vi "Oxford-1820-Main_.vi"() -> ()   [LabVIEW 2016]
uses:
  <instrlib>/Mercury iXX/Public/Controls/Unit String.ctl
  <instrlib>/Mercury iXX/Public/Libraries/Temperature/Controls/Temperature Device (Read).ctl
  <instrlib>/Mercury iXX/Public/Controls/Manufacturing Data.ctl
  <instrlib>/Mercury iXX/Public/Libraries/Temperature/Controls/Temperature Sensor Type.ctl
  <instrlib>/Mercury iXX/Public/Libraries/Temperature/Controls/Excitation Cluster.ctl
  <instrlib>/Mercury iXX/Public/Libraries/Temperature/Controls/Excitation Type.ctl
  <instrlib>/Mercury iXX/Public/Libraries/Temperature/Controls/Calibration Cluster.ctl
  <instrlib>/Mercury iXX/Public/Libraries/Temperature/Controls/Calibration Interpolation.ctl
  <instrlib>/Mercury iXX/Public/Libraries/Temperature/Controls/Loop Cluster.ctl
  <instrlib>/Mercury iXX/Public/Libraries/Temperature/Controls/Temperature Signals Cluster.ctl
  <instrlib>/Mercury iXX/Public/Libraries/Heater/Controls/Heater Device (Read).ctl
  <instrlib>/Mercury iXX/Public/Libraries/Heater/Controls/Heater Signals Cluster.ctl
  <instrlib>/Mercury iXX/Public/Libraries/Level Meter/Controls/Level Meter (Read).ctl
  <instrlib>/Mercury iXX/Public/Libraries/Level Meter/Controls/Nitrogen Configuration.ctl
  <instrlib>/Mercury iXX/Public/Libraries/Level Meter/Controls/Frequency Configuration.ctl
  <instrlib>/Mercury iXX/Public/Libraries/Level Meter/Controls/Signals.ctl
  <instrlib>/Mercury iXX/Public/Libraries/Level Meter/Controls/Helium Configuration.ctl
  <instrlib>/Mercury iXX/Public/Libraries/Level Meter/Controls/Resistance Configuration.ctl
  <instrlib>/Mercury iXX/Public/Libraries/Level Meter/Controls/Pre-Pulse.ctl
  <instrlib>/Mercury iXX/Public/Libraries/Level Meter/Controls/Pulse.ctl
  <instrlib>/Mercury iXX/Public/Libraries/Auxiliary/Controls/AUX Device (Read).ctl
  <instrlib>/Mercury iXX/Public/Libraries/Auxiliary/Controls/AUX Signals (Read).ctl
  <instrlib>/Mercury iXX/Public/Libraries/Magnet/Controls/Device (Read).ctl
  <instrlib>/Mercury iXX/Public/Libraries/Magnet/Controls/Signals (Read).ctl
  <instrlib>/Mercury iXX/Public/Libraries/Magnet/Controls/Identifier.ctl
  <instrlib>/Mercury iXX/Public/Libraries/Pressure/Controls/Pressure Device (Read).ctl
  <instrlib>/Mercury iXX/Public/Libraries/Pressure/Controls/Pressure Sensor Type.ctl
  <instrlib>/Mercury iXX/Public/Libraries/Pressure/Controls/Calibration Cluster.ctl
  <instrlib>/Mercury iXX/Public/Libraries/Pressure/Controls/Calibration Interpolation.ctl
  <instrlib>/Mercury iXX/Public/Libraries/Pressure/Controls/Loop Cluster.ctl
  <instrlib>/Mercury iXX/Public/Libraries/Pressure/Controls/Pressure Signals Cluster.ctl
  <instrlib>/Mercury iXX/Mercury iXX.lvlib
  <instrlib>/Mercury iXX/Public/Controls/Comms Transport Layer.ctl
  <instrlib>/Mercury iXX/Public/Libraries/Pressure/Open/Open Pressure Device.vi
  <instrlib>/Mercury iXX/Public/Libraries/Pressure.lvlib
  <instrlib>/Mercury iXX/Public/Libraries/Pressure/Configuration/Read/Pressure Device (Read).vi
  <instrlib>/Mercury iXX/Public/Libraries/System/Read/Display Automatic Dimming (Read).vi
  <instrlib>/Mercury iXX/Public/Libraries/System.lvlib
  <instrlib>/Mercury iXX/Public/Libraries/System/Read/Display Automatic Dimming Time (Read).vi
  <instrlib>/Mercury iXX/Public/Libraries/System/Read/Display Brightness (Read).vi
  <instrlib>/Mercury iXX/Public/Libraries/System/Read/Mode (Read).vi
  <instrlib>/Mercury iXX/Public/Libraries/System/Read/Serial Number (Read).vi
  <instrlib>/Mercury iXX/Public/Libraries/System/Read/FVer (Read).vi
  <instrlib>/Mercury iXX/Public/Libraries/System/Read/HVer (Read).vi
  <instrlib>/Mercury iXX/Public/Libraries/System/Set/DateTime (Set).vi
  <instrlib>/Mercury iXX/Public/Libraries/Control Loop/Configuration/Read/Control Loop (Read).vi
  <instrlib>/Mercury iXX/Public/Libraries/Control Loop.lvlib
  <instrlib>/Mercury iXX/Public/Libraries/Heater/Configuration/Read/Maximum Power (Read).vi
  <instrlib>/Mercury iXX/Public/Libraries/Heater.lvlib
  <instrlib>/Mercury iXX/Public/Libraries/Heater/Configuration/Read/Nominal Resistance (Read).vi
  <instrlib>/Mercury iXX/Public/Libraries/Temperature/Signals/Read/Temperature (Read).vi
  <instrlib>/Mercury iXX/Public/Libraries/Temperature.lvlib
  <instrlib>/Mercury iXX/Public/Libraries/Pressure/Signals/Read/Current (Read).vi
  <instrlib>/Mercury iXX/Public/Libraries/Temperature/Configuration/Read/Calibration Cold Limit (Read).vi
  <instrlib>/Mercury iXX/Public/Libraries/Temperature/Configuration/Read/Calibration Hot Limit (Read).vi
  <instrlib>/Mercury iXX/Public/Libraries/Temperature/Configuration/Read/Excitation Type (Read).vi
  <instrlib>/Mercury iXX/Public/Libraries/Temperature/Configuration/Read/Temperature Sensor (Read).vi
  <instrlib>/Mercury iXX/Public/Libraries/Temperature/Configuration/Read/Temperature Device (Read).vi
  <instrlib>/Mercury iXX/Public/Libraries/Temperature/Configuration/Read/Nickname (Read).vi
  <instrlib>/Mercury iXX/Public/Libraries/Temperature/Configuration/Read/Excitation Magnitude (Read).vi
  <instrlib>/Mercury iXX/Public/Libraries/Temperature/Configuration/Read/Serial Number (Read).vi
  <instrlib>/Mercury iXX/Public/Libraries/System/Read/Catalogue (Read).vi
  <instrlib>/Mercury iXX/Public/Libraries/System/Read/Flash Space (Read).vi
  <instrlib>/Mercury iXX/Public/Libraries/System/Read/DateTime (Read).vi
  <instrlib>/Mercury iXX/Public/Libraries/System/Read/Time (Read).vi
  <instrlib>/Mercury iXX/Public/Libraries/System/Read/Date (Read).vi
  <instrlib>/Mercury iXX/Public/Libraries/System/Open/Open System.vi
  <instrlib>/Mercury iXX/Public/Libraries/Temperature/Open/Open Temperature Device.vi
  <instrlib>/Mercury iXX/Public/Libraries/Pressure/Signals/Read/Voltage (Read).vi
  <instrlib>/Mercury iXX/Public/Libraries/Auxiliary/Open/Open Auxiliary Device.vi
  <instrlib>/Mercury iXX/Public/Libraries/Auxiliary.lvlib
  <instrlib>/Mercury iXX/Public/Libraries/Auxiliary/Signals/Read/Percent Open (Read).vi
  <instrlib>/Mercury iXX/Public/Libraries/Auxiliary/Configuration/Read/Temperature Error Sensitivity (Read).vi
  <instrlib>/Mercury iXX/Public/Libraries/Auxiliary/Configuration/Read/Valve Gearing (Read).vi
  <instrlib>/Mercury iXX/Public/Libraries/Auxiliary/Configuration/Read/Temperature Error Voltage Sensitivity (Read).vi
  <instrlib>/Mercury iXX/Public/Libraries/Magnet/Configuration/Read/Current to Field Factor (Read).vi
  <instrlib>/Mercury iXX/Public/Libraries/Magnet.lvlib
  <instrlib>/Mercury iXX/Public/Libraries/Magnet/Open/Open Magnet Device.vi
  <instrlib>/Mercury iXX/Public/Libraries/Magnet/Configuration/Read/PSU Action Status (Read).vi
  <instrlib>/Mercury iXX/Public/Libraries/Magnet/Configuration/Read/Magnet Device (Read).vi
  <instrlib>/Mercury iXX/Public/Libraries/Magnet/Configuration/Read/Switch Present (Read).vi
  <instrlib>/Mercury iXX/Public/Libraries/Temperature/Signals/Read/Voltage (Read).vi
  <instrlib>/Mercury iXX/Private/Controls/Query Dynamic Reference.ctl
  <instrlib>/Mercury iXX/Public/Controls/Mercury Reference.ctl
  <instrlib>/Mercury iXX/Public/Libraries/Level Meter/Open/Open Level Meter Device.vi
  <instrlib>/Mercury iXX/Public/Libraries/Level Meter.lvlib
  <instrlib>/Mercury iXX/Public/Libraries/Level Meter/Signals/Read/Probe Level Nitrogen (Read).vi
  <instrlib>/Mercury iXX/Public/Libraries/Level Meter/Configuration/Read/Nitrogen Freq at 100 (Read).vi
  <instrlib>/Mercury iXX/Public/Libraries/Level Meter/Signals/Read/Probe Level Helium (Read).vi
  <instrlib>/Mercury iXX/Public/Libraries/Level Meter/Signals/Read/Probe Resistance Helium (Read).vi
  <instrlib>/Mercury iXX/Public/Libraries/Level Meter/Configuration/Read/Nitrogen Pulse Count Period (Read).vi
  <instrlib>/Mercury iXX/Public/Libraries/Magnet/Signals/Read/Switch Heater Status (Read).vi
  <instrlib>/Mercury iXX/Public/Libraries/Magnet/Signals/Read/Current (Read).vi
  <instrlib>/Mercury iXX/Public/Libraries/Magnet/Configuration/Set/PSU Action Status (Set).vi
  <instrlib>/Mercury iXX/Public/Libraries/Magnet/Controls/PSU Actions.ctl
  <instrlib>/Mercury iXX/Public/Libraries/Magnet/Signals/Set/Target Field Rate (Set).vi
  <instrlib>/Mercury iXX/Public/Libraries/Magnet/Signals/Read/Persistant Field (Read).vi
  <instrlib>/Mercury iXX/Public/Libraries/Magnet/Signals/Read/Target Field (Read).vi
  <instrlib>/Mercury iXX/Public/Libraries/Magnet/Signals/Set/Target Field (Set).vi
  <instrlib>/Mercury iXX/Public/Libraries/Magnet/Configuration/Read/Software Voltage Limit (Read).vi
  <instrlib>/Mercury iXX/Public/Controls/ISOBus Address.ctl
  <instrlib>/Mercury iXX/Public/Libraries/Heater/Signals/Read/Power (Read).vi
  <instrlib>/Mercury iXX/Public/Libraries/Heater/Signals/Read/Voltage (Read).vi
  <instrlib>/Mercury iXX/Public/Libraries/Auxiliary/Signals/Read/Position (Read).vi
  <instrlib>/Mercury iXX/Public/Libraries/Auxiliary/Configuration/Read/Stepper Speed (Read).vi
  <instrlib>/Mercury iXX/Public/Libraries/Level Meter/Signals/Read/Probe Count Nitrogen (Read).vi
  <instrlib>/Mercury iXX/Public/Libraries/Magnet/Signals/Read/Current Rate (Read).vi
  <instrlib>/Mercury iXX/Public/Libraries/Lambda/Configuration/Set/Lambda Percentage Flow (Set).vi
  <instrlib>/Mercury iXX/Public/Libraries/Lambda.lvlib
  <instrlib>/Mercury iXX/Public/Libraries/Lambda/Open/Open Lambda Device.vi
  <instrlib>/Mercury iXX/Public/Libraries/Lambda/Configuration/Set/Lambda Flow Auto (Set).vi
  <instrlib>/Mercury iXX/Public/Libraries/Level Meter/Configuration/Set/Pulse Slow-Fast (Set).vi
  <instrlib>/Mercury iXX/Public/Controls/Response String.ctl
  <instrlib>/Mercury iXX/Public/Libraries/Temperature/Signals/Read/Resistance (Read).vi
  <instrlib>/Mercury iXX/Public/Libraries/Magnet/Signals/Read/Persistant Current (Read).vi
  <userlib>/_OpenG.lib/error/error.llb/Filter Error Codes (Array)__ogtk.vi
  <instrlib>/Mercury iXX/Public/Libraries/Heater/Configuration/Read/Nickname (Read).vi
  <instrlib>/Mercury iXX/Public/Libraries/Heater/Configuration/Read/Voltage Limit (Read).vi
  <instrlib>/Mercury iXX/Public/Libraries/Heater/Configuration/Read/Serial Number (Read).vi
  <instrlib>/Mercury iXX/Public/Libraries/Heater/Configuration/Read/Heater Device (Read).vi
  <instrlib>/Mercury iXX/Public/Libraries/Heater/Open/Open Heater Device.vi
  <instrlib>/Mercury iXX/Public/Libraries/Auxiliary/Configuration/Read/Gas Flow Scaling (Read).vi
  <instrlib>/Mercury iXX/Public/Libraries/Auxiliary/Configuration/Read/Minimum Gas Flow (Read).vi
  <instrlib>/Mercury iXX/Public/Libraries/Auxiliary/Configuration/Read/Serial Number (Read).vi
  <instrlib>/Mercury iXX/Public/Libraries/Auxiliary/Configuration/Read/Aux Device (Read).vi
  <instrlib>/Mercury iXX/Public/Libraries/Pressure/Configuration/Read/Nickname (Read).vi
  <instrlib>/Mercury iXX/Public/Libraries/Level Meter/Configuration/Read/Helium Pulse Duration (Read).vi
  <instrlib>/Mercury iXX/Public/Libraries/Level Meter/Configuration/Read/Helium Pulse Mag (Read).vi
  <instrlib>/Mercury iXX/Public/Libraries/Level Meter/Configuration/Read/Helium Probe Resistance (Read).vi
  <instrlib>/Mercury iXX/Public/Libraries/Level Meter/Configuration/Read/Serial Number (Read).vi
  <instrlib>/Mercury iXX/Public/Libraries/Level Meter/Configuration/Read/Level Meter Device (Read).vi
  <instrlib>/Mercury iXX/Public/Libraries/Magnet/Configuration/Read/Current Limit (Read).vi
  <instrlib>/Mercury iXX/Public/Libraries/Magnet/Configuration/Read/Output Configuration (Read).vi
  <instrlib>/Mercury iXX/Public/Libraries/Magnet/Configuration/Read/Bipolar Output (Read).vi
  <instrlib>/Mercury iXX/Public/Libraries/Magnet/Configuration/Read/Serial Number (Read).vi
  <instrlib>/Mercury iXX/Public/Libraries/Magnet/Signals/Read/Target Field Rate (Read).vi
  <instrlib>/Mercury iXX/Public/Libraries/Magnet/Signals/Read/Field (Read).vi
  <instrlib>/Mercury iXX/Public/Libraries/Magnet/Signals/Read/Voltage (Read).vi
  <instrlib>/Mercury iXX/Public/Libraries/Heater/Signals/Read/Current (Read).vi
  <instrlib>/Mercury iXX/Public/Libraries/Magnet/Controls/Switch Heater.ctl
  <instrlib>/Mercury iXX/Public/Libraries/Magnet/Signals/Set/Switch Heater Status (Set).vi
panel:
  in  "Tab Control 6":enum32{"Page 1", "Page 2"}(tab)
  in  "Tab Control 5":enum32{"Page 1", "Page 2"}(tab)
  in  "Open Needle Valve":bool
  in  "Close Needle Valve":bool
  in  "Lambda":bool
  out "LPF NV (%)":dbl format="%_6g"
  out "LPF Pressure":dbl format="%_5f mB"
  out "Magnet Field (T) 2":dbl(knob) caption="Voltage (V)" scale=-20.0..20.0
  out "Voltage (V) 2":dbl(knob)=-0.0003 caption="Voltage (V)" scale=-10.0..10.0
  out "Current (A)":dbl(knob)=0.0006 scale=-180.0..180.0
  in  "Tab Control 4":enum32{"Page 1", "Page 2"}(tab)
  out "N2 LEVEL":dbl=61.3025 format="%.0f %"
  out "He LVL Chart":dbl(slide)=52.0833 scale=0.0..100.0
  out "N2 LVL Chart":dbl(slide)=61.3025 scale=0.0..100.0
  out "He LEVEL 3":dbl=61.3025 format="%.0f %"
  in  "Fast/Slow Fill":bool
  in  "Tab Control 3":enum32{"Page 1", "Page 2"}(tab)
  out "Magnet T":dbl=3.8705 format="%_2f K"
  out "Magnet R":dbl=3.8705 format="%_3f ohms"
  out "LPF R":dbl=4.2075 format="%_3f ohms"
  out "Voltage (V)":dbl=-0.0003 format="%.5f"
  out "LPF T":dbl=4.2075 format="%_2f K"
  out "Current (A)":dbl=0.0006 format="%.5f"
  out "Magnet Status 2":string
  in  "Tab Control 2":enum32{"Page 1", "Page 2"}(tab)
  in  "Hold":bool
  in  "To Set":bool
  in  "Send to IPS":bool
  out "Power Supply Field (T)":dbl=0.0001 format="%#.5f"
  in  "Target Field (T) 2":dbl format="%#.5f"
  out "Target Field (T)":dbl format="%#.5f"
  in  "Target Rate (T/min)":dbl=0.1 format="%.5f"
  out "Target  Rate (T/min)":dbl=1.0 format="%.5f"
  out "Magnet Field (T)":dbl format="%.5f"
  out "He LEVEL":dbl=52.0833 format="%.0f %"
  in  "PS Heat":bool
  out "Switch Time":string="11:11:48"
  in  "To Zero":bool
  in  "Clamp":bool
  in  "Toolbar":enum32{"Page 1", "Page 2"}(tab)
  in  "Start 2":bool
  in  "Stop 2":bool
  in  "Minimize":bool
  out "ETA":string
  out "Magnet Status 3":string="Clamped"
  in  "Remote Mode":bool
  out "Sentinel":bool=TRUE
  out "SWITCH HEATER":bool
  out "LPF ON":timestamp
  in  "Tab Control":T1(tab)
  in  "Mercury Functions":T2(tab)=enum."Temperature"
  out "time stamp":timestamp=timestamp(3543841780 s since 1904-01-01)
  out "Free Space":i32=166384 caption="Free Space (KB)"
  out "Set Date Response":string="VALID"
  out "String":string="NORM" caption="User Mode"
  out "Date":string="2016:04:18"
  out "Time":string="11:29:40"
  out "Hardware Version":string="65"
  out "Firmware Version":string="2.2.6.20"
  out "Serial Number":string="154650110"
  out "ITC Devices":string[](array[string])=["DB4.G1:AUX", "DB8.P1:PRES", "MB0.H1:HTR", "MB1.T1:TEMP"]
  out "S/W Version(s)":string[](array[string])=["2.2.6.20\n"]
  out "Serial Number(s)":string[](array[string])=["154650110"]
  out "# of Instruments":i32=1
  out "Automatic Dimming":string="OFF"
  out "Dimming Time":string="5"
  out "Display Brightness":string="100"
  in  "ITC IP Address":string="130.49.180.101"
  out "Excitation Magnitude":dbl=5.0
  out "Sensor Type":string="NTC"
  out "Excitation Type":string="UNIP"
  out "Hot Limit":dbl=1000.0
  out "H Unit":T3="K"
  out "Cold Limit":dbl=1000.0
  out "C Unit":T3="K"
  out "Unit":T3
  out "Voltage":dbl=0.005
  out "V Unit":T3="V"
  out "Temperature":dbl=4.2075
  out "T Unit":T3="K"
  out "Temperature Device Settings":T4={"Manufacturing"={"Hardware Version"="65", "Firmware Version"="2.2", "Serial Number"="154650110"}, "Temperature Sensor Type"="NTC", "Excitation"={"Excitation Type"="UNIP", "Magnitude"="5.00"}, "Calibration"={"Filename"="59543_iTC-lambda.dat", "Interpolation"="LIN", "Scaling Factor"="1", "Offset Factor"="0", "Hot Limit"="1000.00K", "Cold Limit"="1000.00K", "Last Calibration"="", "Reference"="Internal"}, "Control Loop"={"Heater"="", "Auxiliary"="", "Heater Auto"="", "Percentage Heat"="", "Temperature Set Point"="", "PID Auto (from file)"="", "P Value"="", "I Value"="", "D Value"="", "Auto PID Table Filename"="", "Flow Auto"="", "Target Heater Table"="", "Sweep mode"="", "Sweep Table Filename"="", "Percentage Flow"=""}, "Temperature Signals"={"Voltage"="5.0000mV", "Current"="3.9694µA", "Power"="0.0199µW", "Resistance"="1259.6510R", "Temperature"="4.2075K", "Sensitivity"="299.3801R/K", "Reference"="N/A"}, "Nickname"="Mag_AB_MB1", "Status"="0"}
  out "Temp S/N":string="154650110"
  out "T Nickname":string="Mag_AB_MB1"
  out "T Loop Details":T11
  out "Heater Device Settings":T13={"Manufacturing"={"Hardware Version"="65", "Firmware Version"="2.3", "Serial Number"="154650110"}, "Nickname"="MB0.H1", "Voltage Limit"="1", "Nominal Resistance"="10", "Maximum Power"="0.1000", "Heater Signals"={"Voltage"="0.0507V", "Current"="-0.0000A", "Power"="0.0000W"}, "Status"="2"}
  out "Htr C Unit":T3="A"
  out "Htr P Unit":T3="W"
  out "Htr V Unit":T3="V"
  out "Htr Current":dbl=-0.0
  out "Htr Power":dbl
  out "Htr Voltage":dbl=0.0507
  out "Power Unit":T3
  out "Volt Unit":T3
  out "Res Unit":T3
  out "Maximum Power":dbl=0.1
  out "Htr Resistance":dbl=10.0
  out "Htr Voltage Limit":dbl=1.0
  out "Htr S/N":string="154650110"
  out "Htr Nickname":string="MB0.H1"
  out "Pressure Device":T15={"Manufacturing"={"Hardware Version"="3", "Firmware Version"="1.10", "Serial Number"="151150091"}, "Temperature Sensor Type"="RAT", "Calibration"={"Filename"="Lambda pressure control_10V ratiometric.dat", "Interpolation"="LIN", "Scaling Factor"="1", "Offset Factor"="-0.0004", "High Limit"="1000.00K", "Low Limit"="1000.00K", "Last Calibration"=""}, "Control Loop"={"Heater"="None", "Auxiliary"="None", "Heater Auto"="", "Percentage Heat"="", "Pressure Set Point"="", "PID Auto (from file)"="", "P Value"="", "I Value"="", "D Value"="1.0", "Auto PID Table Filename"="", "Flow Auto"="", "Target Heater Table"="", "Sweep mode"="", "Sweep Table Filename"="", "Percentage Flow"=""}, "Pressure Signals"={"Voltage"="-0.0822mV", "Current"="-0.0000A", "Power"="0.0000W", "Pressure"="0.0000mB"}, "Nickname"="Lam_P_DB8", "Status"="0"}
  out "Nickname":string="Lam_P_DB8"
  out "Current":dbl=-0.0
  out "Voltage":dbl=-8.219999999999999e-05
  out "Auxiliary Device Details":T21={"Manufacturing"={"Hardware Version"="65", "Firmware Version"="3.1", "Serial Number"="154650084"}, "Min Flow"=0.0, "Scaling Factor"=50.0, "Temp Err"=9.0, "Temp V Err"=11.0, "Gear"=2, "Speed"=2, "Signals"={"Position"=0.0, "% Open"=0.0, "I0"="ON", "I1"="OFF", "I2"="OFF", "I3"="OFF", "O0"="OFF", "O1"="OFF", "O2"="OFF", "O3"="OFF"}, "Nickname"="DB4.G1", "Status"="0"} {"Signals"."% Open" min=0.0 max=100.0 step=0.1 format="%.4f"; "Signals"."Position" max=20.0 step=1.0 format="%.4f"; "Speed" max=7 step=1; "Gear" max=7 step=1; "Temp V Err" min=0.0 max=20.0 step=0.1; "Temp Err" min=0.0 max=20.0 step=0.1; "Scaling Factor" min=0.0 max=99.0 step=0.1; "Min Flow" min=0.0 max=20.0 step=0.1}
  out "Aux S/N":string="154650084"
  out "Min Flow":dbl caption="Minimum Gas Flow" format="%#.1f"
  out "Scaling Factor":dbl=50.0 caption="Gas Flow Scaling Factor" format="%#.1f"
  out "Temp Err":dbl=9.0 caption="Temperature Error Sensitivity" format="%#.1f"
  out "Temp V Err":dbl=11.0 caption="Temperature Voltage Error Sensitivity" format="%#.1f"
  out "Gear":u32=2 caption="Valve Gearing"
  out "Speed":u32=2 caption="Stepper Speed"
  out "Unit 2":T3
  out "Unit 3":T3
  out "Unit 4":T3
  out "Unit 5":T3
  out "Unit 6":T3
  out "Unit 7":T3
  out "Position":u32
  out "% Open":dbl caption="Percentage Open (%)"
  out "Unit":T3
  out "Unit":T3="%"
  out "time stamp 2":timestamp=timestamp(3543841781 s since 1904-01-01)
  out "Free Space 2":i32=166316 caption="Free Space (KB)"
  out "Set Date Response 2":string="VALID"
  out "String 2":string="NORM" caption="User Mode"
  out "Date 2":string="2016:04:18"
  out "Time 2":string="11:29:45"
  out "Hardware Version 2":string="65"
  out "Firmware Version 2":string="2.2.6.20"
  out "Serial Number 2":string="153350063"
  out "IPS Devices":string[](array[string])=["DB3.L1:LVL", "GRPX:PSU", "GRPY:PSU", "GRPZ:PSU", "MB1.T1:TEMP", "PSU.M1:PSU", "PSU.M2:PSU", "PSU.M3:PSU"]
  out "S/W Version(s) 2":string[](array[string])=["2.2.6.20\n"]
  out "Serial Number(s) 2":string[](array[string])=["153350063"]
  out "# of Instruments 2":i32=1
  out "Automatic Dimming 2":string="OFF"
  out "Dimming Time 2":string="5"
  out "Display Brightness 2":string="100"
  in  "IPS IP Address":string="130.49.180.102"
  out "LVL Device DetailSettings":T23={"Manufacturing"={"Hardware Version"="65", "Firmware Version"="2.2", "Serial Number"="152450013"}, "Nitrogen Configuration"={"Frequency Configuration"={"Freq 0%"=0.0, "Freq 100%"=0.0}, "Pulse Period"=0.0}, "Signals"={"Helium Signals"={"Resistance"=75.5626, "Level"=52.0833}, "Nitrogen Signals"={"Count"=8800.0, "Freq"=487361.0, "Level"=61.3445}}, "Nickname"="DB3.L1", "Status"="0", "Helium Configuration"={"Resistance Configuration"={"Res 0%"=0.0, "Res 100%"=0.0}, "Pre-Pulse"={"Magnitude"=0.0, "Duration"=0.0}, "Pulse"={"Magnitude"=0.0, "Duration"=0.0, "Delay"=0.0}}}
  out "LVL S/N":string="152450013"
  out "LVL P Magnitude":dbl=125.0 caption="Pulse Magnitude (mA)"
  out "LVL P Duration":dbl=5.0 caption="Pulse Duration (s)"
  out "N Freq 100%":dbl=7880.0 caption="Frequency at 100% (Hz)"
  out "N Pulse Period":dbl=1000.0 caption="Pulse Period (ms)"
  out "He Res Config":T28={"Res 0%"=149.0, "Res 100%"=8.0}
  out "He Resistance":dbl=75.5626 caption="Resistance (Ohms)"
  out "He Level":dbl=52.0833 caption="Helium Level (%)"
  out "N Counter":u32 caption="Counter"
  out "N Level":dbl=61.3445 caption="Nitrogen Level (%)"
  out "Excitation Magnitude 2":dbl=5.0
  out "Sensor Type 2":string="NTC"
  out "Excitation Type 2":string="UNIP"
  out "Hot Limit 2":dbl=1000.0
  out "H Unit 2":T3="K"
  out "Cold Limit 2":dbl=1000.0
  out "C Unit 2":T3="K"
  out "Unit 12":T3
  out "Voltage 2":dbl=0.005
  out "V Unit 2":T3="V"
  out "Temperature 2":dbl=3.8706
  out "T Unit 2":T3="K"
  out "Temperature Device Settings 2":T4={"Manufacturing"={"Hardware Version"="65", "Firmware Version"="2.2", "Serial Number"="153350063"}, "Temperature Sensor Type"="NTC", "Excitation"={"Excitation Type"="UNIP", "Magnitude"="5.00"}, "Calibration"={"Filename"="Bob.dat", "Interpolation"="LIN", "Scaling Factor"="1", "Offset Factor"="0", "Hot Limit"="1000.00K", "Cold Limit"="1000.00K", "Last Calibration"="", "Reference"="Internal"}, "Control Loop"={"Heater"="", "Auxiliary"="", "Heater Auto"="", "Percentage Heat"="", "Temperature Set Point"="", "PID Auto (from file)"="", "P Value"="", "I Value"="", "D Value"="", "Auto PID Table Filename"="", "Flow Auto"="", "Target Heater Table"="", "Sweep mode"="", "Sweep Table Filename"="", "Percentage Flow"=""}, "Temperature Signals"={"Voltage"="5.0000mV", "Current"="3.5897µA", "Power"="0.0179µW", "Resistance"="1392.8897R", "Temperature"="3.8706K", "Sensitivity"="359.8580R/K", "Reference"="N/A"}, "Nickname"="MB1.T1", "Status"="0"}
  out "Temp S/N 2":string="153350063"
  out "T Nickname 2":string="MB1.T1"
  out "T Loop Details 2":T11
  out "Magnet Device Details":T31={"Manufacturing"={"Hardware Version"="NOT_FOUND", "Firmware Version"="NOT_FOUND", "Serial Number"="NOT_FOUND"}, "Nickname"="GRPZ", "Bipolar Output"="ON", "String"="PARA", "Current Limit"=174.0, "AtoB"=8.688, "Inductance"=39.406, "Switch Present"="PSU.M1", "Swh Htr Current"=86.0, "SW VLIM"=9.0, "V Trans Time"=1000.0, "Magnet PSU Signals"={"Voltage"=-0.0002, "Current"=0.0002, "Current Rate"=100.0, "Field"=0.0001, "Field Rate"=11.5101, "Persistant Current"=0.0003, "Persistant Field"=0.0, "Target Current"=0.0, "Target Field"=0.0, "Target Current Rate"=8.688, "Target Field Rate"=1.0, "Switch Heater Status (SWHT)"="OFF", "Switch Heater Status (SWHN)"="OFF"}, "PSU Action"="CLMP", "Status"="40000000", "Level Limit"=0.0, "Temperature Limit"=999.0} {"Temperature Limit" format="%#.1f"; "Level Limit" format="%#.1f"; "V Trans Time" format="%#.1f"; "SW VLIM" format="%#.1f"; "Swh Htr Current" format="%#.1f"; "Inductance" format="%#.1f"; "AtoB" format="%#.1f"; "Current Limit" format="%#.1f"}
  out "Mag S/N":string="NOT_FOUND"
  out "Bipolar Output":string="ON"
  out "Out Config":string="PARA" caption="Output Configuration"
  out "Current Limit":dbl=174.0 caption="Current Limit (A)" format="%#.1f"
  out "AtoB":dbl=8.688 caption="Current Field Factor (A/T)" format="%#.1f"
  out "Switch Present":string="PSU.M1"
  out "SW VLIM":dbl=9.0 caption="Software Voltage Limit (V)" format="%#.1f"
  out "Unit 8":T3
  out "Unit 9":T3
  out "Unit 10":T3
  out "Current Rate":dbl=100.0
  out "PSU Act Stat":string="CLMP" caption="PSU Action Status"
  out "Unit 11":T3="A/min"
  in  "Device Identifier":T33="GRPZ"
  out "Error List":T34(array[cluster])
  out "LPF on (s)":i32=5373
  # "Magnet (T)"
  # "Voltage (V)"
  # "Current (A)"
  # "Slow Rates\nCurrent Range (A)     Field Range (T)   Rate (T/min)\n0       -- 100        0    -- 11.5      0.91\n100     -- 150        11.5 -- 17.2      0.23\n150     -- 155.467    17.2 -- 18        0.11\n155.567 -- 172.471    18   -- 20        0.11\n\nFast Rates\nCurrent Range (A)     Field Range (T)   Rate (T/min)\n0       -- 155.467    0    -- 18        1.0\n155.567 -- 172.471    18   -- 20        0.25"
  # "Helium"
  # "Nitrogen"
  # "v17/02/01"
  # "ITC: 101\nIPS: 102\nIPS VR: 67"
  # "ITC: 101\nIPS: 102\nIPS VR: 67"
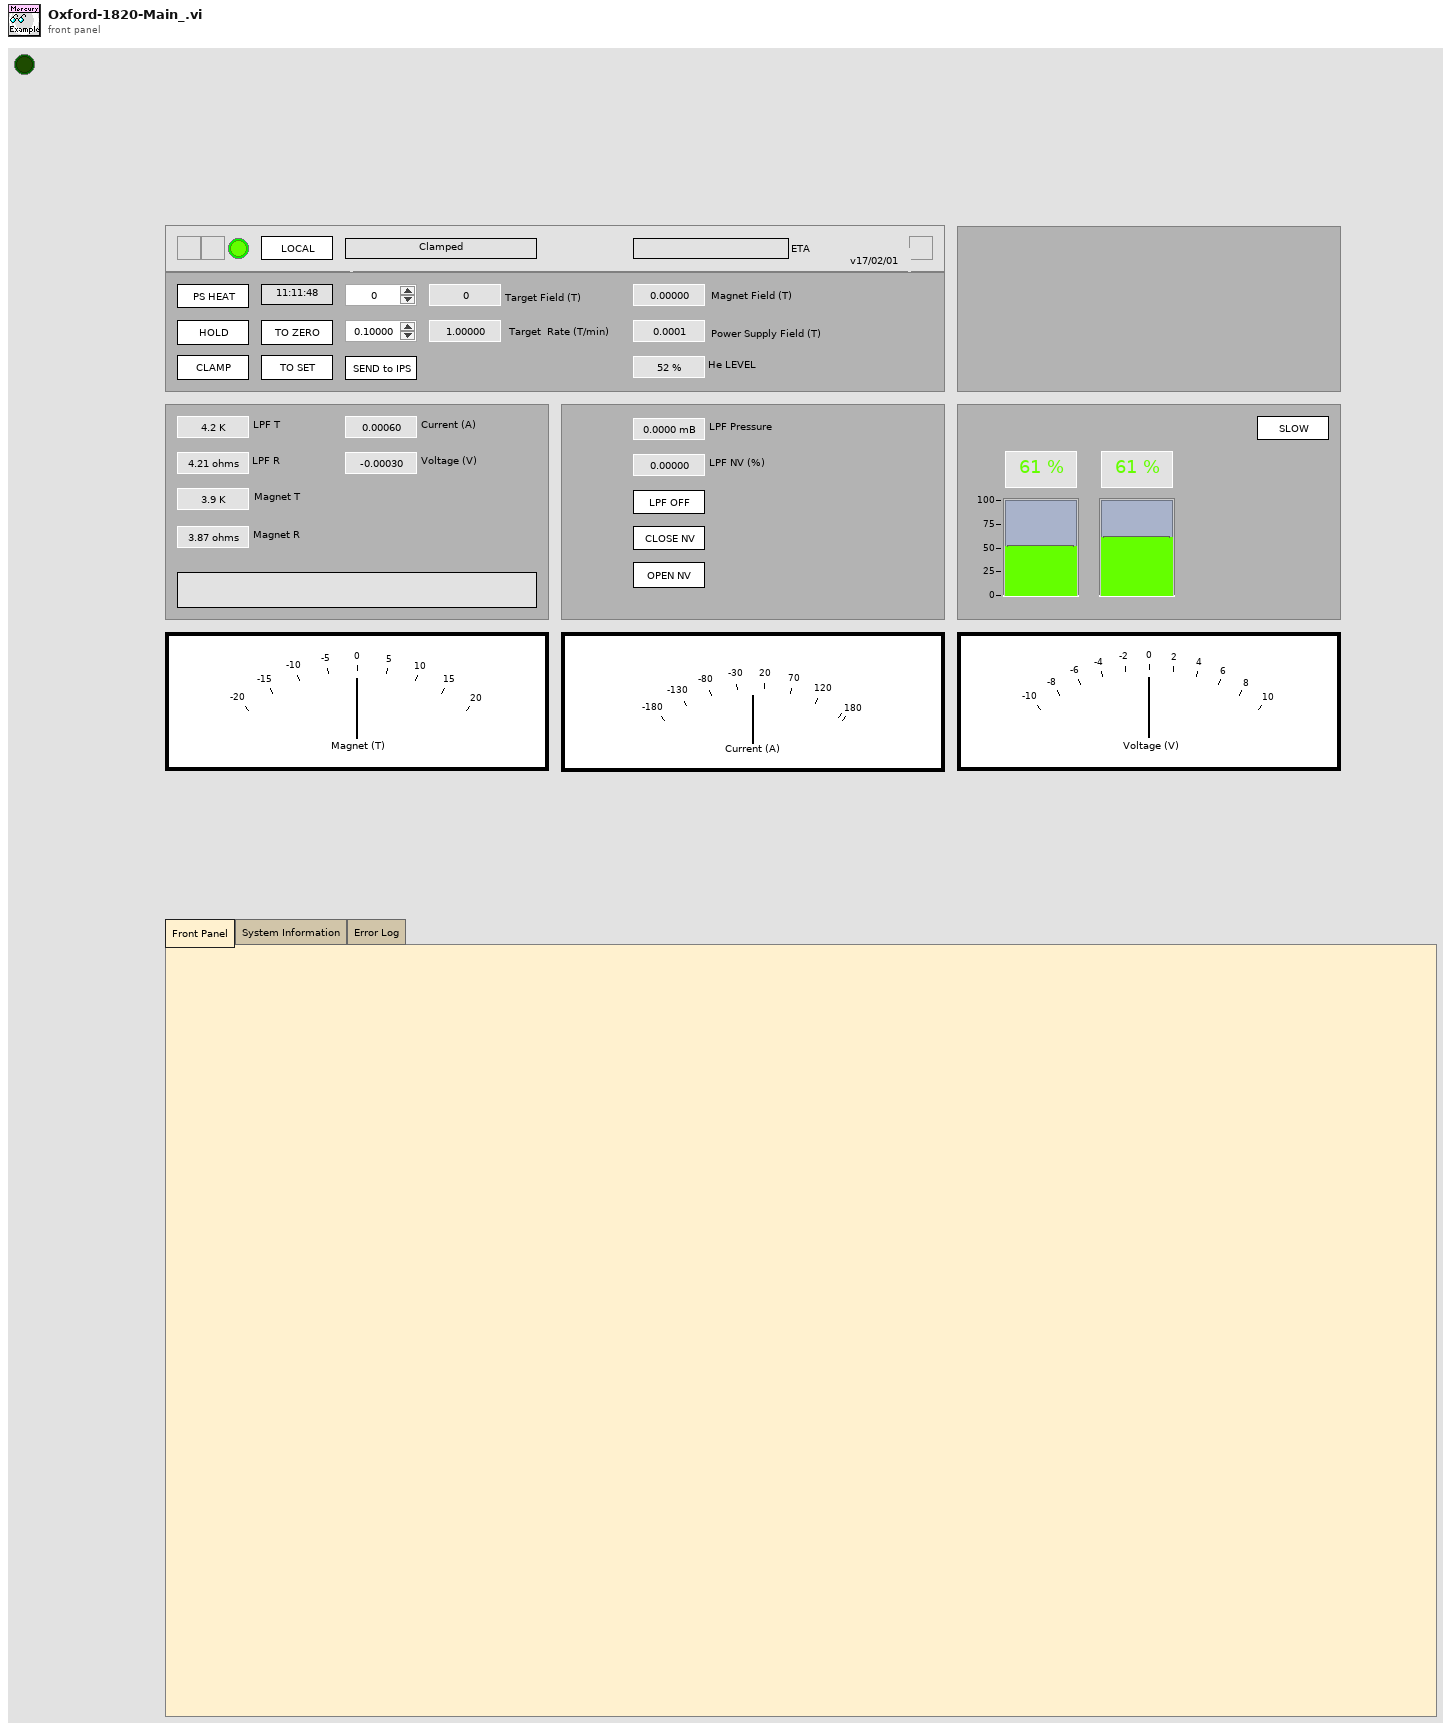
[diagram p1: front panel]
types:
  T1 = enum32{"Front Panel", "System Information", "Error Log"}
  T2 = enum32{"System: ITC", "Temperature", "Heater", "Pressure", "Auxiliary", "System: IPS", "Level Meter", "Temperature 2", "Magnet"}
  T3 = typedef "Mercury iXX.lvlib/Unit String.ctl" = string
  T4 = typedef "Mercury iXX.lvlib/Temperature.lvlib/Temperature Device (Read).ctl" = cluster{"Manufacturing":T5, "Temperature Sensor Type":T6, "Excitation":T7, "Calibration":T9, "Control Loop":T11, "Temperature Signals":T12, "Nickname":string, "Status":string}
  T5 = typedef "Mercury iXX.lvlib/Manufacturing Data.ctl" = cluster{"Hardware Version":string, "Firmware Version":string, "Serial Number":string}
  T6 = typedef "Mercury iXX.lvlib/Temperature.lvlib/Temperature Sensor Type.ctl" = string
  T7 = typedef "Mercury iXX.lvlib/Temperature.lvlib/Excitation Cluster.ctl" = cluster{"Excitation Type":T8, "Magnitude":string}
  T8 = typedef "Mercury iXX.lvlib/Temperature.lvlib/Excitation Type.ctl" = string
  T9 = typedef "Mercury iXX.lvlib/Temperature.lvlib/Calibration Cluster.ctl" = cluster{"Filename":string, "Interpolation":T10, "Scaling Factor":string, "Offset Factor":string, "Hot Limit":string, "Cold Limit":string, "Last Calibration":string, "Reference":string}
  T10 = typedef "Mercury iXX.lvlib/Temperature.lvlib/Calibration Interpolation.ctl" = string
  T11 = typedef "Mercury iXX.lvlib/Temperature.lvlib/Loop Cluster.ctl" = cluster{"Heater":string, "Auxiliary":string, "Heater Auto":string, "Percentage Heat":string, "Temperature Set Point":string, "PID Auto (from file)":string, "P Value":string, "I Value":string, "D Value":string, "Auto PID Table Filename":string, "Flow Auto":string, "Target Heater Table":string, "Sweep mode":string, "Sweep Table Filename":string, "Percentage Flow":string}
  T12 = typedef "Mercury iXX.lvlib/Temperature.lvlib/Temperature Signals Cluster.ctl" = cluster{"Voltage":string, "Current":string, "Power":string, "Resistance":string, "Temperature":string, "Sensitivity":string, "Reference":string}
  T13 = typedef "Mercury iXX.lvlib/Heater.lvlib/Heater Device (Read).ctl" = cluster{"Manufacturing":T5, "Nickname":string, "Voltage Limit":string, "Nominal Resistance":string, "Maximum Power":string, "Heater Signals":T14, "Status":string}
  T14 = typedef "Mercury iXX.lvlib/Heater.lvlib/Heater Signals Cluster.ctl" = cluster{"Voltage":string, "Current":string, "Power":string}
  T15 = typedef "Mercury iXX.lvlib/Pressure.lvlib/Pressure Device (Read).ctl" = cluster{"Manufacturing":T5, "Temperature Sensor Type":T16, "Calibration":T17, "Control Loop":T19, "Pressure Signals":T20, "Nickname":string, "Status":string}
  T16 = typedef "Mercury iXX.lvlib/Pressure.lvlib/Pressure Sensor Type.ctl" = string
  T17 = typedef "Mercury iXX.lvlib/Pressure.lvlib/Calibration Cluster.ctl" = cluster{"Filename":string, "Interpolation":T18, "Scaling Factor":string, "Offset Factor":string, "High Limit":string, "Low Limit":string, "Last Calibration":string}
  T18 = typedef "Mercury iXX.lvlib/Pressure.lvlib/Calibration Interpolation.ctl" = string
  T19 = typedef "Mercury iXX.lvlib/Pressure.lvlib/Loop Cluster.ctl" = cluster{"Heater":string, "Auxiliary":string, "Heater Auto":string, "Percentage Heat":string, "Pressure Set Point":string, "PID Auto (from file)":string, "P Value":string, "I Value":string, "D Value":string, "Auto PID Table Filename":string, "Flow Auto":string, "Target Heater Table":string, "Sweep mode":string, "Sweep Table Filename":string, "Percentage Flow":string}
  T20 = typedef "Mercury iXX.lvlib/Pressure.lvlib/Pressure Signals Cluster.ctl" = cluster{"Voltage":string, "Current":string, "Power":string, "Pressure":string}
  T21 = typedef "Mercury iXX.lvlib/Auxiliary.lvlib/AUX Device (Read).ctl" = cluster{"Manufacturing":T5, "Min Flow":dbl, "Scaling Factor":dbl, "Temp Err":dbl, "Temp V Err":dbl, "Gear":u32, "Speed":u32, "Signals":T22, "Nickname":string, "Status":string}
  T22 = typedef "Mercury iXX.lvlib/Auxiliary.lvlib/AUX Signals (Read).ctl" = cluster{"Position":dbl, "% Open":dbl, "I0":string, "I1":string, "I2":string, "I3":string, "O0":string, "O1":string, "O2":string, "O3":string}
  T23 = typedef "Mercury iXX.lvlib/Level Meter.lvlib/Level Meter (Read).ctl" = cluster{"Manufacturing":T5, "Nitrogen Configuration":T24, "Signals":T26, "Nickname":string, "Status":string, "Helium Configuration":T27}
  T24 = typedef "Mercury iXX.lvlib/Level Meter.lvlib/Nitrogen Configuration.ctl" = cluster{"Frequency Configuration":T25, "Pulse Period":dbl}
  T25 = typedef "Mercury iXX.lvlib/Level Meter.lvlib/Frequency Configuration.ctl" = cluster{"Freq 0%":dbl, "Freq 100%":dbl}
  T26 = typedef "Mercury iXX.lvlib/Level Meter.lvlib/Signals.ctl" = cluster{"Helium Signals":cluster{"Resistance":dbl, "Level":dbl}, "Nitrogen Signals":cluster{"Count":dbl, "Freq":dbl, "Level":dbl}}
  T27 = typedef "Mercury iXX.lvlib/Level Meter.lvlib/Helium Configuration.ctl" = cluster{"Resistance Configuration":T28, "Pre-Pulse":T29, "Pulse":T30}
  T28 = typedef "Mercury iXX.lvlib/Level Meter.lvlib/Resistance Configuration.ctl" = cluster{"Res 0%":dbl, "Res 100%":dbl}
  T29 = typedef "Mercury iXX.lvlib/Level Meter.lvlib/Pre-Pulse.ctl" = cluster{"Magnitude":dbl, "Duration":dbl}
  T30 = typedef "Mercury iXX.lvlib/Level Meter.lvlib/Pulse.ctl" = cluster{"Magnitude":dbl, "Duration":dbl, "Delay":dbl}
  T31 = typedef "Mercury iXX.lvlib/Magnet.lvlib/Device (Read).ctl" = cluster{"Manufacturing":T5, "Nickname":string, "Bipolar Output":string, "String":string, "Current Limit":dbl, "AtoB":dbl, "Inductance":dbl, "Switch Present":string, "Swh Htr Current":dbl, "SW VLIM":dbl, "V Trans Time":dbl, "Magnet PSU Signals":T32, "PSU Action":string, "Status":string, "Level Limit":dbl, "Temperature Limit":dbl}
  T32 = typedef "Mercury iXX.lvlib/Magnet.lvlib/Signals (Read).ctl" = cluster{"Voltage":dbl, "Current":dbl, "Current Rate":dbl, "Field":dbl, "Field Rate":dbl, "Persistant Current":dbl, "Persistant Field":dbl, "Target Current":dbl, "Target Field":dbl, "Target Current Rate":dbl, "Target Field Rate":dbl, "Switch Heater Status (SWHT)":string, "Switch Heater Status (SWHN)":string}
  T33 = typedef "Mercury iXX.lvlib/Magnet.lvlib/Identifier.ctl" = string
  T34 = cluster{"time":timestamp, "code":i32, "source":string}[]
  T35 = typedef "LVRectTypeDef.ctl" = cluster{"Left":i16, "Top":i16, "Right":i16, "Bottom":i16}
  T36 = cluster{"Hold":bool, "Clamp":bool, "To Set":bool, "To Zero":bool, "Send to IPS":bool, "PS Heat":bool, "Lambda":bool}
  T37 = typedef "Mercury iXX.lvlib/Magnet.lvlib/PSU Actions.ctl" = string
  T38 = typedef "Mercury iXX.lvlib/Magnet.lvlib/Switch Heater.ctl" = string
  T39 = typedef "Mercury iXX.lvlib/ISOBus Address.ctl" = i32
  T40 = typedef "Mercury iXX.lvlib/Response String.ctl" = string
  T41 = enum32{"invalid app kind", "Development System", "Run Time System", "Student Edition", "Embedded LabVIEW", "Evaluation", "Custom"}
  T42 = cluster{"time":timestamp, "code":i32, "source":string}
  T43 = enum32{"Invalid", "Standard", "Closed", "Hidden", "Minimized", "Maximized"}
  T44 = cluster{"Magnet Field":dbl, "PS Field":dbl, "Target Field":dbl, "Target Field Rate":dbl, "Voltage":dbl, "Current":dbl}
  T45 = typedef "Mercury iXX.lvlib/Comms Transport Layer.ctl" = enum16{"Ethernet TCP/IP", "USB", "ISOBus - RS-232", "GPIB"}
  T46 = typedef "Mercury iXX.lvlib/Query Dynamic Reference.ctl" = refnum<vi>
  T47 = typedef "Mercury iXX.lvlib/Mercury Reference.ctl" = cluster{"Comms":refnum<visa-resource-name>, "Device ID":string[], "Comms Layer":T45, "Command":string, "Query reference":T46}
  T48 = cluster{"Core":cluster{"Current VI Reference":refnum<vi>, "Close Panel on Exit?":bool}, "Mercury ITC Ref":cluster{"Comms":refnum<visa-resource-name>, "Device ID":string[], "Comms Layer":T45, "Command":string, "Query reference":T46}, "Mercury IPS Ref":T47, "sentinel":bool, "Error Log":cluster{"time":timestamp, "code":i32, "source":string}[]}
  T49 = typedef "Actions.ctl" = cluster{"Hold":bool, "Clamp":bool, "To Set":bool, "To Zero":bool, "Send to IPS":bool, "PS Heat":bool, "Lambda":bool}
  T50 = typedef "Targets.ctl" = cluster{"Target Field (T)":dbl, "Target Field Rate (T/min)":dbl}
  T51 = cluster{"Target Field (T)":dbl, "Target Field Rate (T/min)":dbl}
  T52 = cluster{"Comms":refnum<visa-resource-name>, "Device ID":string[], "Comms Layer":T45, "Command":string, "Query reference":T46}
  T53 = typedef "Filtered Error Details - Cluster__ogtk.ctl" = cluster{"code":i32, "source":string}
  T54 = cluster{"Current VI Reference":refnum<vi>, "Close Panel on Exit?":bool}
  T55 = typedef "Mercury iXX.lvlib/System.lvlib/User Mode.ctl" = string
  T56 = typedef "Mercury iXX.lvlib/Magnet.lvlib/Output Configuration.ctl" = string
  T57 = typedef "Status.ctl" = cluster{"Magnet Field":dbl, "PS Field":dbl, "Target Field":dbl, "Target Field Rate":dbl, "Voltage":dbl, "Current":dbl, "Switch":bool, "Mercury State":string}
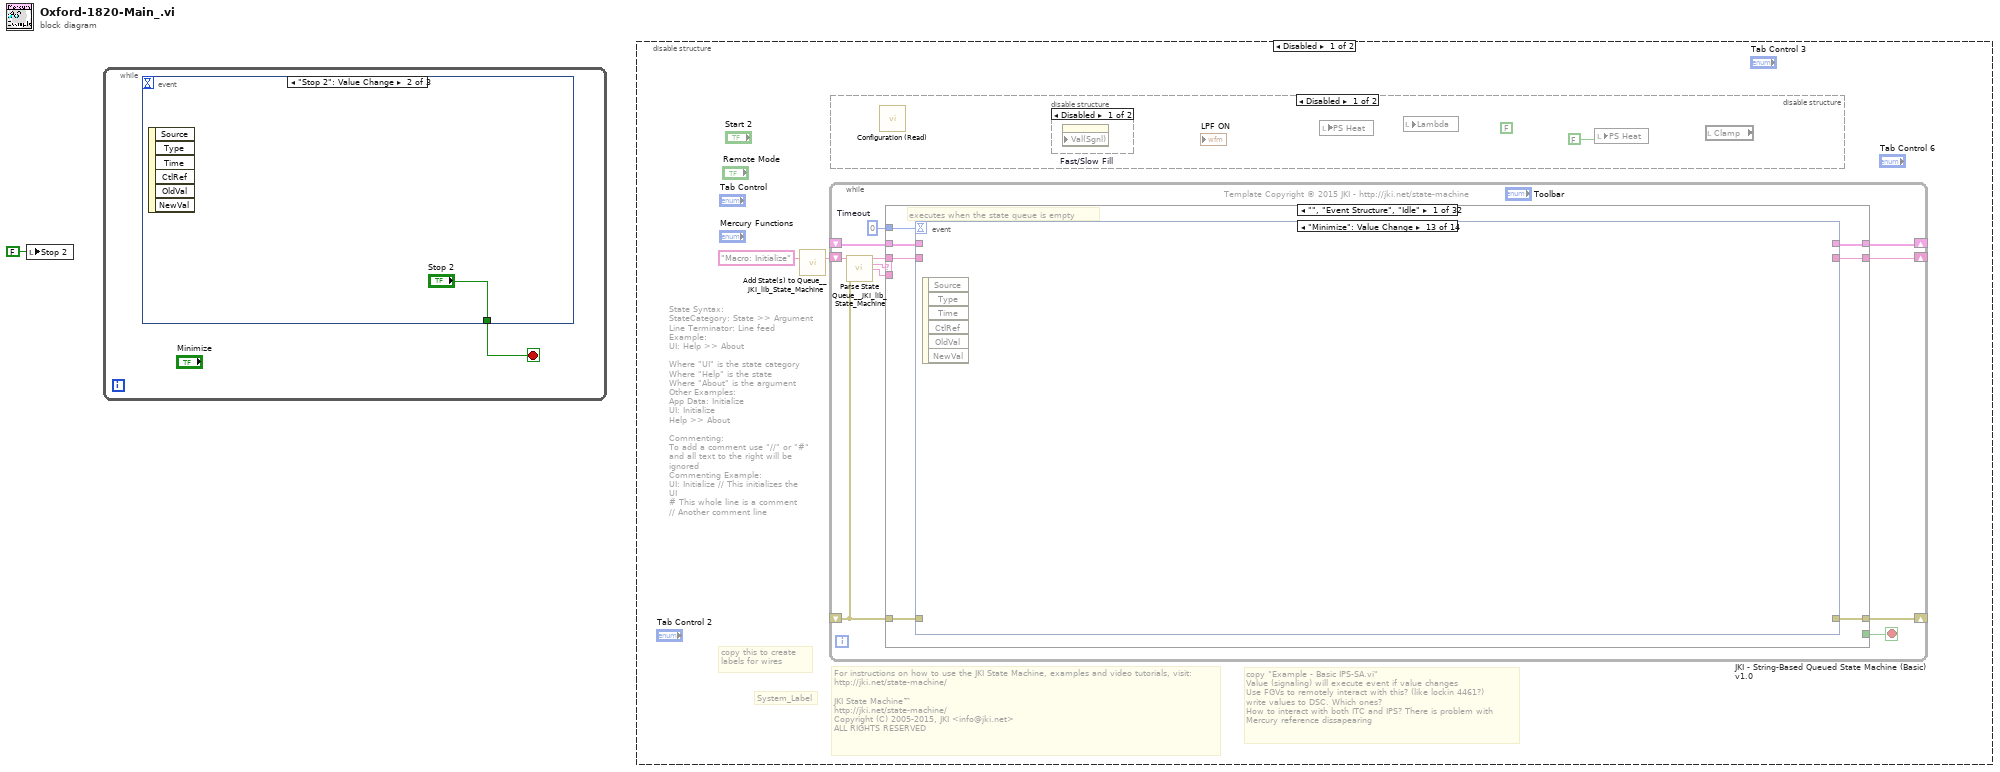
[diagram p0: block diagram]
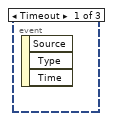
[diagram p2: hidden frame]
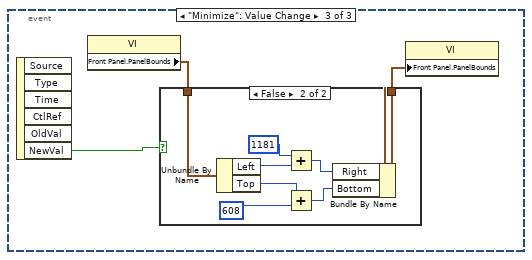
[diagram p3: hidden frame]
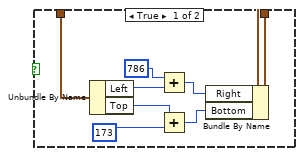
[diagram p4: hidden frame]
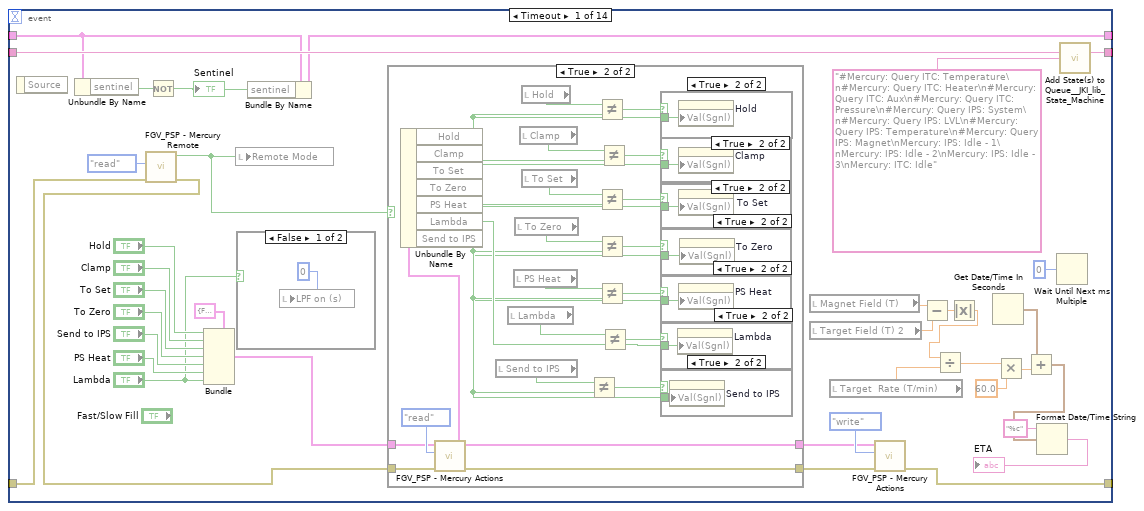
[diagram p7: hidden frame]
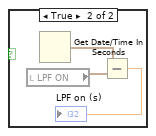
[diagram p8: hidden frame]
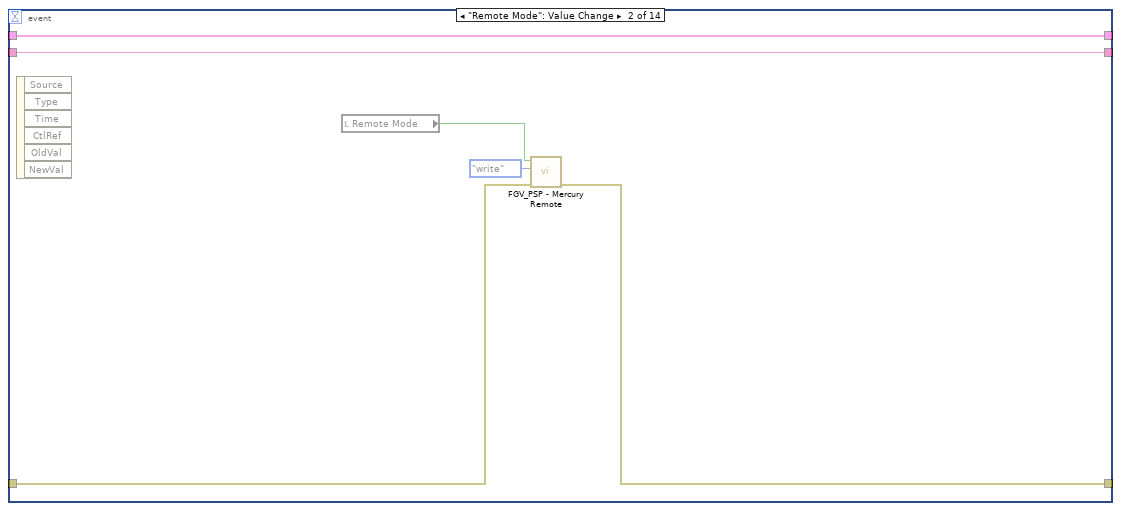
[diagram p17: hidden frame]
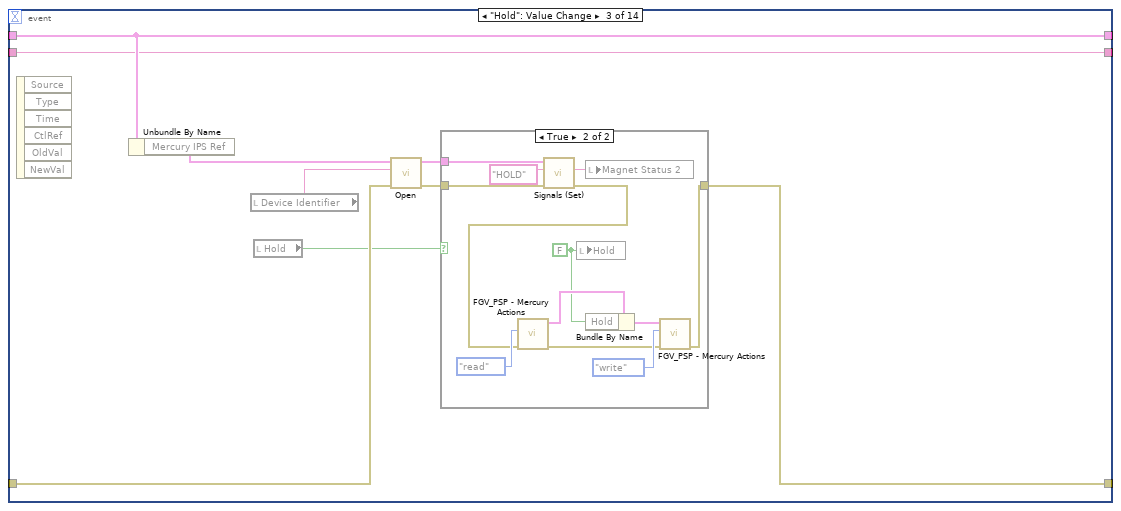
[diagram p18: hidden frame]
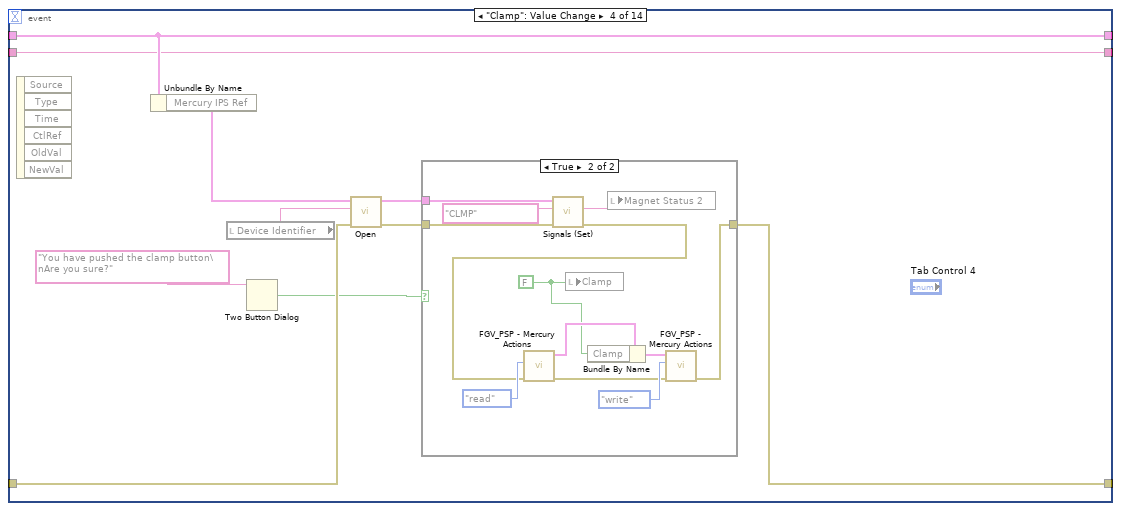
[diagram p20: hidden frame]
diagram:
  n1 = local write "Stop 2"(FALSE ("Stop 2")) -> ()
  n2 = while {
    stop <- w2 stop-if-true
    n3 = event shown="[1] \"Stop 2\": Value Change" {
      selector: _ -> [_ _ _]
      dyn-events: _ -> [_ _ _]
      timeout: _ -> [_ _ _]
      tunnel: [_ "Stop 2" _] -> w2
      event Timeout {
        n4 = event-data() -> ()  [unwired: 1 in, 3 out]
      }
      event "Stop 2": Value Change {
        n5 = event-data() -> ()  [unwired: 1 in, 6 out]
      }
      event "Minimize": Value Change {
        n6 = event-data() -> ("NewVal"=w4:bool)  [unwired: 1 in, 5 out]
        n7 = property class="VI"() -> ("Front Panel.PanelBounds"=w6:T35)  [unwired: 2 in, 2 out]
        n8 = case shown="False" w4 {
          tunnel: w6 -> [w14 w22]
          tunnel: [w13 w21] -> w5
          frame True {
            n9 = Unbundle By Name(w14) -> ("Left"=w12:i16, "Top"=w10:i16)
            n10 = Add(x=i16 786 ("x 6"), y=w12) -> (x+y=w11:i16)
            n11 = Add(x=w10, y=i16 173 ("x 5")) -> (x+y=w9:i16)
            n12 = Bundle By Name(cluster=w14, "Right"=w11, "Bottom"=w9) -> (w13:T35)
          }
          frame False {
            n13 = Unbundle By Name(w22) -> ("Left"=w20:i16, "Top"=w18:i16)
            n14 = Add(x=i16 1181 ("x 8"), y=w20) -> (x+y=w19:i16)
            n15 = Add(x=w18, y=i16 608 ("x 7")) -> (x+y=w17:i16)
            n16 = Bundle By Name(cluster=w22, "Right"=w19, "Bottom"=w17) -> (w21:T35)
          }
        }
        n17 = property class="VI"("Front Panel.PanelBounds"=w5) -> ()  [unwired: 2 in, 2 out]
      }
    }
  }
  n18 = disable-structure shown="Disabled" {
    frame Disabled {
      # "copy \"Example - Basic IPS-SA.vi\"\nValue (signaling) will execute event if value changes\nUse FGVs to remotely interact with this? (like lockin 4461?)\nwrite values to DSC. Which ones?\nHow to interact with both ITC and IPS? There is problem with \nMercury reference dissapearing"
      # "For instructions on how to use the JKI State Machine, examples and video tutorials, visit:\nhttp://jki.net/state-machine/\n\nJKI State Machine™\nhttp://jki.net/state-machine/\nCopyright (C) 2005-2015, JKI <info@jki.net>\nALL RIGHTS RESERVED"
      # "State Syntax:\nStateCategory: State >> Argument\nLine Terminator: Line feed\nExample:\nUI: Help >> About\n\nWhere \"UI\" is the state category\nWhere \"Help\" is the state\nWhere \"About\" is the argument\nOther Examples:\nApp Data: Initialize\nUI: Initialize\nHelp >> About\n\nCommenting:\nTo add a comment use \"//\" or \"#\" and all text to the right will be ignored\nCommenting Example:\nUI: Initialize // This initializes the UI\n# This whole line is a comment\n// Another comment line"
      # "copy this to create labels for wires"
      # "System_Label"
      n19 = call <vilib>:"Add State(s) to Queue__JKI_lib_State_Machine.vi"("State(s) in (\"\")"="Macro: Initialize") -> ("States Out"=w24:string)  [unwired: 14 in]
      n20 = while "JKI - String-Based Queued State Machine (Basic) v1.0" {
        shift-right: [w29] -> _
        shift-left: _ -> [w28]
        shift-right: [w32] -> _
        shift-left: _ -> [w26]
        shift-right: [w31] -> _
        shift-left: w24 -> [w33]
        stop <- w30 stop-if-true
        w27 = 0  # Timeout
        # "Template Copyright © 2015 JKI - http://jki.net/state-machine"
        n21 = call <vilib>:"Parse State Queue__JKI_lib_State_Machine.vi"("State Queue"=w33, "Error In (no error)"=w26) -> ("Remaining States"=w35:string, "Current State"=w36:string, "Arguments"=w34:string)  [unwired: 11 in]
        n22 = case shown="\"\", \"Event Structure\", \"Idle\"" w36 {
          selector: w36 -> [_ _ w373 _ _ _ _ _ _ _ _ _ _ _ _ _ _ _ _ _ _ _ _ _ _ _ _ _ _ _ _ _]
          tunnel: w35 -> [w43 w372 w377 w395 w412 w417 w421 w430 w436 w440 w452 w459 w470 w496 w501 w516 w520 w543 w587 w633 w675 w722 w743 w788 w829 w876 w917 w960 w1020 w1062 w1066 w1071]
          tunnel: w34 -> [_ _ _ _ _ _ _ _ _ _ _ w454 w464 _ _ _ _ _ _ _ _ _ _ _ _ _ _ _ _ _ _ _]
          tunnel: w28 -> [w39 w369 w375 w386 w398 w415 w418 _ w431 w437 w450 w457 w466 w493 w499 w514 w517 w538 w585 w632 w639 w682 w729 w786 w828 w875 w916 w959 w1019 w1061 w1065 w1070]
          tunnel: [w37 w370 w379 w392 errorcluster {"status"=FALSE, "code"=0, "source"=""} ("error out") w414 w419 w423 w432 w438 w446 w455 w467 w494 w498 w502 w518 w522 w547 w594 w636 w685 w730 w750 w795 w834 w883 w922 w998 w1036 w1064 w1068] -> w32
          tunnel: [w42 w371 w376 w394 w411 w416 w420 w429 w435 w439 w451 w458 w469 w495 w500 w515 w519 w542 w586 w634 w676 w723 w744 w787 w830 w877 w918 w961 w1021 w1063 w1067 w1072] -> w31
          tunnel: [_ _ _ _ _ TRUE _ _ _ _ _ _ _ _ _ _ _ _ _ _ _ _ _ _ _ _ _ _ _ _ _ _] -> w30
          tunnel: [w41 w369 w375 w393 w397 w415 w418 w428 w431 w437 w450 w457 w466 w493 w499 w514 w517 w537 w585 w632 w639 w682 w729 w786 w828 w875 w916 w959 w1019 w1061 w1065 w1070] -> w29
          tunnel: w27 -> [w40 _ _ _ _ _ _ _ _ _ _ _ _ _ _ _ _ _ _ _ _ _ _ _ _ _ _ _ _ _ _ _]
          tunnel: w26 -> [w38 w370 w378 w392 w407 w414 w419 w423 w433 w438 w442 w456 w468 w494 w498 w504 w518 w530 w549 w595 w642 w684 w724 w752 w797 w831 w878 w958 w999 w1037 w1064 w1069]
          frame "", "Event Structure", "Idle" {
            # "executes when the state queue is empty"
            n23 = event shown="[12] \"Minimize\": Value Change" {
              selector: _ -> [_ _ _ _ _ _ _ _ _ _ _ _ _ _]
              dyn-events: _ -> [_ _ _ _ _ _ _ _ _ _ _ _ _ _]
              timeout: w40 -> [_ _ _ _ _ _ _ _ _ _ _ _ _ _]
              tunnel: w43 -> [w80 w122 w133 w156 w177 w200 w225 w268 w307 w326 w337 w362 _ w368]
              tunnel: [w79 w122 w133 w156 w177 w200 w225 w268 w307 w326 w337 w361 _ w367] -> w42
              tunnel: [w74 w121 w134 w157 w178 w199 w226 w264 w306 w320 w339 w359 _ w365] -> w41
              tunnel: w39 -> [w75 w121 w134 w157 w178 w199 w226 w264 w306 w320 w339 w359 _ w365]
              tunnel: w38 -> [w58 w124 w130 w152 w172 w194 w220 w267 w304 w324 w338 w360 _ w366]
              tunnel: [w68 w123 w132 w150 w179 w201 w224 w265 w298 w311 w330 w360 _ w366] -> w37
              event Timeout {
                n24 = event-data() -> ()  [unwired: 1 in, 1 out]
                n25 = Unbundle By Name(w75) -> ("sentinel"=w77:bool)
                n26 = call "FGV_PSP - Mercury Remote.vi"("error in"=w58, "Function"=enum16{"write", "read"}."read") -> ("error out"=w57:errorcluster, "Remote"=w56:bool)  [unwired: 4 in]
                n27 = Not(x=w77) -> (.not. x?=w76:bool)
                "Sentinel" <- w76
                n28 = Bundle(cluster=T36 {"Hold"=FALSE, "Clamp"=FALSE, "To Set"=FALSE, "To Zero"=FALSE, "Send to IPS"=FALSE, "PS Heat"=FALSE, "Lambda"=FALSE}, "Hold"="Hold", "Clamp"="Clamp", "To Set"="To Set", "To Zero"="To Zero", "Send to IPS"="Send to IPS", "PS Heat"="PS Heat", "Lambda"="Lambda") -> (w66:T36)
                n29 = local write "Remote Mode"(w56) -> ()
                n30 = case shown="False" "Lambda" {
                  frame False {
                    n31 = local write "LPF on (s)"(0 ("LPF on (s)")) -> ()
                  }
                  frame True {
                    n32 = local read "LPF ON"() -> (w84:timestamp)
                    n33 = Get Date/Time In Seconds() -> (seconds since 1Jan1904=w83:timestamp)
                    n34 = Subtract(x=w83, y=w84) -> (x-y=→"LPF on (s)":dbl)
                  }
                }
                n35 = Bundle By Name(cluster=w75, "sentinel"=w76) -> (w74:T48)
                n36 = case shown="True" w56 {
                  tunnel: [w85 w111] -> w67
                  tunnel: w57 -> [w85 w110]
                  tunnel: w66 -> [w86 w109]
                  tunnel: [w86 w101] -> w65
                  frame False {
                  }
                  frame True {
                    n37 = call "FGV_PSP - Mercury Actions.vi"("error in"=w110, "Function"=enum16{"write", "read"}."read", "Actions"=w109) -> ("error out"=w111:errorcluster, "Actions"=w101:T49)  [unwired: 3 in]
                    n38 = Unbundle By Name(w101) -> ("Hold"=w93:bool, "Clamp"=w95:bool, "To Set"=w96:bool, "To Zero"=w97:bool, "PS Heat"=w98:bool, "Lambda"=w99:bool, "Send to IPS"=w100:bool)
                    n39 = local read "Send to IPS"() -> (w94:bool)
                    n40 = local read "Lambda"() -> (w92:bool)
                    n41 = local read "PS Heat"() -> (w91:bool)
                    n42 = local read "To Zero"() -> (w90:bool)
                    n43 = local read "Clamp"() -> (w88:bool)
                    n44 = local read "Hold"() -> (w87:bool)
                    n45 = local read "To Set"() -> (w89:bool)
                    n46 = Not Equal?(x=w94, y=w100) -> (x != y?=w102:bool)
                    n47 = Not Equal?(x=w87, y=w93) -> (x != y?=w108:bool)
                    n48 = Not Equal?(x=w89, y=w96) -> (x != y?=w106:bool)
                    n49 = Not Equal?(x=w90, y=w97) -> (x != y?=w105:bool)
                    n50 = Not Equal?(x=w91, y=w98) -> (x != y?=w104:bool)
                    n51 = Not Equal?(x=w88, y=w95) -> (x != y?=w107:bool)
                    n52 = Not Equal?(x=w92, y=w99) -> (x != y?=w103:bool)
                    n53 = case shown="True" w108 {
                      tunnel: w93 -> [_ w119]
                      frame False {
                      }
                      frame True {
                        n54 = property on="Hold" class="Bool (strict)"("Val(Sgnl)"=w119) -> ()  [unwired: 2 in, 2 out]
                      }
                    }
                    n55 = case shown="True" w107 {
                      tunnel: w95 -> [_ w118]
                      frame False {
                      }
                      frame True {
                        n56 = property on="Clamp" class="Bool (strict)"("Val(Sgnl)"=w118) -> ()  [unwired: 2 in, 2 out]
                      }
                    }
                    n57 = case shown="True" w106 {
                      tunnel: w96 -> [_ w117]
                      frame False {
                      }
                      frame True {
                        n58 = property on="To Set" class="Bool (strict)"("Val(Sgnl)"=w117) -> ()  [unwired: 2 in, 2 out]
                      }
                    }
                    n59 = case shown="True" w105 {
                      tunnel: w97 -> [_ w116]
                      frame False {
                      }
                      frame True {
                        n60 = property on="To Zero" class="Bool (strict)"("Val(Sgnl)"=w116) -> ()  [unwired: 2 in, 2 out]
                      }
                    }
                    n61 = case shown="True" w104 {
                      tunnel: w98 -> [_ w115]
                      frame False {
                      }
                      frame True {
                        n62 = property on="PS Heat" class="Bool (strict)"("Val(Sgnl)"=w115) -> ()  [unwired: 2 in, 2 out]
                      }
                    }
                    n63 = case shown="True" w103 {
                      tunnel: w99 -> [_ w114]
                      frame False {
                      }
                      frame True {
                        n64 = property on="Lambda" class="Bool (strict)"("Val(Sgnl)"=w114) -> ()  [unwired: 2 in, 2 out]
                      }
                    }
                    n65 = case shown="True" w102 {
                      tunnel: w100 -> [_ w113]
                      frame False {
                      }
                      frame True {
                        n66 = property on="Send to IPS" class="Bool (strict)"("Val(Sgnl)"=w113) -> ()  [unwired: 2 in, 2 out]
                      }
                    }
                  }
                }
                n67 = local read "Magnet Field (T)"() -> (w54:dbl)
                n68 = local read "Target Field (T) 2"() -> (w53:dbl)
                n69 = local read "Target  Rate (T/min)"() -> (w55:dbl)
                n70 = call "FGV_PSP - Mercury Actions.vi"("error in"=w67, "Function"=enum16{"write", "read"}."write", "Actions"=w65) -> ("error out"=w68:errorcluster)  [unwired: 3 in, 1 out]
                n71 = Subtract(x=w54, y=w53) -> (x-y=w52:dbl)
                n72 = Absolute Value(x=w52) -> (abs(x)=w51:dbl)
                n73 = Divide(x=w51, y=w55) -> (x/y=w50:dbl)
                n74 = Get Date/Time In Seconds() -> (seconds since 1Jan1904=w47:timestamp)
                n75 = Multiply(x=w50, y=60.0) -> (x*y=w48:dbl)
                n76 = Add(x=w47, y=w48) -> (x+y=w46:timestamp)
                n77 = Format Date/Time String(time format string (%c)="%c", seconds (now)=w46) -> (date/time string=→"ETA":string)  [unwired: 1 in]
                n78 = Wait Until Next ms Multiple(millisecond multiple=u32 0) -> ()  [unwired: 1 out]
                n79 = call <vilib>:"Add State(s) to Queue__JKI_lib_State_Machine.vi"("State(s) in (\"\")"=w80, "State(s) at Back (\"\")"="#Mercury: Query ITC: Temperature\n#Mercury: Query ITC: Heater\n#Mercury: Query ITC: Aux\n#Mercury: Query ITC: Pressure\n#Mercury: Query IPS: System\n#Mercury: Query IPS: LVL\n#Mercury: Query IPS: Temperature\n#Mercury: Query IPS: Magnet\nMercury: IPS: Idle - 1\nMercury: IPS: Idle - 2\nMercury: IPS: Idle - 3\nMercury: ITC: Idle" ("State(s) at Back (\"\")")) -> ("States Out"=w79:string)  [unwired: 13 in]
              }
              event "Remote Mode": Value Change {
                n80 = event-data() -> ()  [unwired: 1 in, 6 out]
                n81 = local read "Remote Mode"() -> (w120:bool)
                n82 = call "FGV_PSP - Mercury Remote.vi"("error in"=w124, "Function"=enum16{"write", "read"}."write", "Remote"=w120) -> ("error out"=w123:errorcluster)  [unwired: 3 in, 1 out]
              }
              event "Hold": Value Change {
                n83 = event-data() -> ()  [unwired: 1 in, 6 out]
                n84 = Unbundle By Name(w134) -> ("Mercury IPS Ref"=w128:T47)
                n85 = local read "Device Identifier"() -> (w129:T33)
                n86 = local read "Hold"() -> (w126:bool)
                n87 = call-poly <instrlib>:"Open.vi"("error in (no error)"=w130, "Device Identifier"=w129, "Mercury Reference In"=w128) -> ("error out"=w131:errorcluster, "Mercury Reference Out"=w127:T47)  [unwired: 7 out]
                n88 = case shown="True" w126 {
                  tunnel: [w135 w137] -> w132
                  tunnel: w131 -> [w135 w146]
                  tunnel: w127 -> [_ w145]
                  frame False {
                  }
                  frame True {
                    w142 = FALSE ("Hold")
                    n89 = call-poly <instrlib>:"Signals (Set).vi"("error in"=w146, "PSU Act Stat"=T37 "HOLD", "Mercury Reference In"=w145) -> ("error out"=w136:errorcluster, "Response"=w144:T40)  [unwired: 1 in, 6 out]
                    n90 = call "FGV_PSP - Mercury Actions.vi"("error in"=w136, "Function"=enum16{"write", "read"}."read") -> ("error out"=w139:errorcluster, "Actions"=w143:T49)  [unwired: 4 in]
                    n91 = local write "Hold"(w142) -> ()
                    n92 = local write "Magnet Status 2"(w144) -> ()
                    n93 = Bundle By Name(cluster=w143, "Hold"=w142) -> (w141:T49)
                    n94 = call "FGV_PSP - Mercury Actions.vi"("error in"=w139, "Function"=enum16{"write", "read"}."write", "Actions"=w141) -> ("error out"=w137:errorcluster)  [unwired: 3 in, 1 out]
                  }
                }
              }
              event "Clamp": Value Change {
                n95 = event-data() -> ()  [unwired: 1 in, 6 out]
                n96 = Unbundle By Name(w157) -> ("Mercury IPS Ref"=w151:T47)
                n97 = local read "Device Identifier"() -> (w155:T33)
                n98 = Two Button Dialog(message="You have pushed the clamp button\nAre you sure?") -> (T button?=w148:bool)  [unwired: 2 in]
                n99 = call-poly <instrlib>:"Open.vi"("error in (no error)"=w152, "Device Identifier"=w155, "Mercury Reference In"=w151) -> ("error out"=w154:errorcluster, "Mercury Reference Out"=w153:T47)  [unwired: 7 out]
                n100 = case shown="True" w148 {
                  tunnel: w154 -> [w158 w168]
                  tunnel: w153 -> [_ w167]
                  tunnel: [w158 w160] -> w150
                  frame False {
                  }
                  frame True {
                    w159 = FALSE
                    n101 = call-poly <instrlib>:"Signals (Set).vi"("error in"=w168, "PSU Act Stat"=T37 "CLMP", "Mercury Reference In"=w167) -> ("error out"=w161:errorcluster, "Response"=w169:T40)  [unwired: 1 in, 6 out]
                    n102 = call "FGV_PSP - Mercury Actions.vi"("error in"=w161, "Function"=enum16{"write", "read"}."read") -> ("error out"=w163:errorcluster, "Actions"=w166:T49)  [unwired: 4 in]
                    n103 = local write "Clamp"(w159) -> ()
                    n104 = Bundle By Name(cluster=w166, "Clamp"=w159) -> (w165:T49)
                    n105 = local write "Magnet Status 2"(w169) -> ()
                    n106 = call "FGV_PSP - Mercury Actions.vi"("error in"=w163, "Function"=enum16{"write", "read"}."write", "Actions"=w165) -> ("error out"=w160:errorcluster)  [unwired: 3 in, 1 out]
                  }
                }
              }
              event "To Set": Value Change {
                n107 = event-data() -> ()  [unwired: 1 in, 6 out]
                n108 = Unbundle By Name(w178) -> ("Mercury IPS Ref"=w174:T47)
                n109 = local read "Device Identifier"() -> (w173:T33)
                n110 = call-poly <instrlib>:"Open.vi"("error in (no error)"=w172, "Device Identifier"=w173, "Mercury Reference In"=w174) -> ("error out"=w175:errorcluster, "Mercury Reference Out"=w176:T47)  [unwired: 7 out]
                n111 = local read "To Set"() -> (w171:bool)
                n112 = case shown="True" w171 {
                  tunnel: [w180 w182] -> w179
                  tunnel: w176 -> [_ w190]
                  tunnel: w175 -> [w180 w189]
                  frame False {
                  }
                  frame True {
                    w181 = FALSE
                    n113 = call-poly <instrlib>:"Signals (Set).vi"("error in"=w189, "PSU Act Stat"=T37 "RTOS", "Mercury Reference In"=w190) -> ("error out"=w183:errorcluster, "Response"=w191:T40)  [unwired: 1 in, 6 out]
                    n114 = call "FGV_PSP - Mercury Actions.vi"("error in"=w183, "Function"=enum16{"write", "read"}."read") -> ("error out"=w185:errorcluster, "Actions"=w188:T49)  [unwired: 4 in]
                    n115 = Bundle By Name(cluster=w188, "To Set"=w181) -> (w187:T49)
                    n116 = local write "To Set"(w181) -> ()
                    n117 = local write "Magnet Status 2"(w191) -> ()
                    n118 = call "FGV_PSP - Mercury Actions.vi"("error in"=w185, "Function"=enum16{"write", "read"}."write", "Actions"=w187) -> ("error out"=w182:errorcluster)  [unwired: 3 in, 1 out]
                  }
                }
              }
              event "To Zero": Value Change {
                n119 = event-data() -> ()  [unwired: 1 in, 6 out]
                n120 = Unbundle By Name(w199) -> ("Mercury IPS Ref"=w196:T47)
                n121 = local read "Device Identifier"() -> (w195:T33)
                n122 = local read "To Zero"() -> (w193:bool)
                n123 = call-poly <instrlib>:"Open.vi"("error in (no error)"=w194, "Device Identifier"=w195, "Mercury Reference In"=w196) -> ("error out"=w197:errorcluster, "Mercury Reference Out"=w198:T47)  [unwired: 7 out]
                n124 = case shown="True" w193 {
                  tunnel: [w202 w205] -> w201
                  tunnel: w198 -> [_ w212]
                  tunnel: w197 -> [w202 w211]
                  frame False {
                  }
                  frame True {
                    w203 = FALSE
                    n125 = call-poly <instrlib>:"Signals (Set).vi"("error in"=w211, "PSU Act Stat"=T37 "RTOZ", "Mercury Reference In"=w212) -> ("error out"=w206:errorcluster, "Response"=w213:T40)  [unwired: 1 in, 6 out]
                    n126 = call "FGV_PSP - Mercury Actions.vi"("error in"=w206, "Function"=enum16{"write", "read"}."read") -> ("error out"=w208:errorcluster, "Actions"=w204:T49)  [unwired: 4 in]
                    n127 = Bundle By Name(cluster=w204, "To Zero"=w203) -> (w210:T49)
                    n128 = local write "To Zero"(w203) -> ()
                    n129 = local write "Magnet Status 2"(w213) -> ()
                    n130 = call "FGV_PSP - Mercury Actions.vi"("error in"=w208, "Function"=enum16{"write", "read"}."write", "Actions"=w210) -> ("error out"=w205:errorcluster)  [unwired: 3 in, 1 out]
                  }
                }
              }
              event "PS Heat": Value Change {
                n131 = event-data() -> ("NewVal"=w215:bool)  [unwired: 1 in, 5 out]
                n132 = local read "Device Identifier"() -> (w221:T33)
                n133 = Unbundle By Name(w226) -> ("Mercury IPS Ref"=w222:T47)
                n134 = call-poly <instrlib>:"Open.vi"("error in (no error)"=w220, "Device Identifier"=w221, "Mercury Reference In"=w222) -> ("error out"=w217:errorcluster, "Mercury Reference Out"=w218:T47)  [unwired: 7 out]
                n135 = call-poly <instrlib>:"Signals (Read).vi"("error in"=w217, "Mercury Reference In"=w218) -> ("error out"=w228:errorcluster, "Current"=w223:dbl, "Mercury Reference Out"=w227:T47)  [unwired: 1 in, 6 out]
                n136 = call-poly <instrlib>:"Signals (Read).vi"("error in"=w228, "Mercury Reference In"=w227) -> ("error out"=w229:errorcluster, "Persistant Current"=w219:dbl, "Mercury Reference Out"=w230:T47)  [unwired: 1 in, 6 out]
                n137 = Subtract(x=w219, y=w223) -> (x-y=w231:dbl)
                n138 = Absolute Value(x=w231) -> (abs(x)=w232:dbl)
                n139 = Less?(x=w232, y=0.1) -> (x < y?=w234:bool)
                n140 = case shown="False" w234 {
                  selector: w234 -> [_ w237]
                  tunnel: [w236 w237] -> w216
                  frame False {
                    n141 = Two Button Dialog(message="The magnet current is more\nthan 0.1A different to the\nPSU output current.  It is not\nadvisable to switch on the\nswitch heater unless these\ncurrents are equal!") -> (T button?=w236:bool)  [unwired: 2 out]
                  }
                  frame True {
                  }
                }
                n142 = case shown="True" w216 {
                  tunnel: w230 -> [_ w257]
                  tunnel: w229 -> [w238 w256]
                  tunnel: [w238 w250] -> w224
                  tunnel: w215 -> [_ w240]
                  frame False {
                  }
                  frame True {
                    n143 = call-poly <instrlib>:"Signals (Read).vi"("error in"=w256, "Mercury Reference In"=w257) -> ("error out"=w245:errorcluster, "Mercury Reference Out"=w241:T47)  [unwired: 1 in, 7 out]
                    n144 = call <userlib>:"Wait (ms)__ogtk.vi"("error in (no error)"=w245, "milliseconds to wait"=u32 100 ("millisecond multiple")) -> ("error out"=w244:errorcluster)  [unwired: 8 in, 1 out]
                    n145 = Select(t=T38 "ON" ("Set Switch Heater"), s=w240, f=T38 "OFF" ("Set Switch Heater")) -> (s? t:f=w242:T38)
                    n146 = call-poly <instrlib>:"Signals (Set).vi"("error in"=w244, "Switch Heater Status"=w242, "Mercury Reference In"=w241) -> ("error out"=w258:errorcluster, "Response"=w247:T40, "Mercury Reference Out"=w259:T47)  [unwired: 1 in, 5 out]
                    n147 = local write "Magnet Status 2"(w247) -> ()
                    n148 = call-poly <instrlib>:"Configuration (Read).vi"("error in"=w258, "Mercury Reference In"=w259) -> ("error out"=w239:errorcluster, "Time"=→"Switch Time":string)  [unwired: 1 in, 7 out]
                    n149 = call "FGV_PSP - Mercury Actions.vi"("error in"=w239, "Function"=enum16{"write", "read"}."read") -> ("error out"=w253:errorcluster, "Actions"=w251:T49)  [unwired: 4 in]
                    n150 = Bundle By Name(cluster=w251, "PS Heat"=w240) -> (w255:T49)
                    n151 = call "FGV_PSP - Mercury Actions.vi"("error in"=w253, "Function"=enum16{"write", "read"}."write", "Actions"=w255) -> ("error out"=w250:errorcluster)  [unwired: 3 in, 1 out]
                  }
                }
              }
              event "Send to IPS": Value Change {
                n152 = event-data() -> ()  [unwired: 1 in, 6 out]
                n153 = local read "Device Identifier"() -> (w263:T33)
                n154 = Unbundle By Name(w264) -> ("Mercury IPS Ref"=w262:T47)
                n155 = local read "Send to IPS"() -> (w260:bool)
                n156 = call-poly <instrlib>:"Open.vi"("error in (no error)"=w267, "Device Identifier"=w263, "Mercury Reference In"=w262) -> ("error out"=w266:errorcluster, "Mercury Reference Out"=w261:T47)  [unwired: 7 out]
                n157 = case shown="True" w260 {
                  tunnel: w266 -> [w269 w288]
                  tunnel: [w269 w272] -> w265
                  tunnel: w261 -> [_ w286]
                  frame False {
                  }
                  frame True {
                    w271 = FALSE
                    n158 = local read "Remote Mode"() -> (w284:bool)
                    n159 = case shown="True" w284 {
                      tunnel: "Target Field (T) 2" -> [w290 _]
                      tunnel: "Target Rate (T/min)" -> [w289 _]
                      tunnel: [w290 w292] -> w278
                      tunnel: [w289 w291] -> w279
                      frame False {
                      }
                      frame True {
                        n160 = call "FGV_PSP - Mercury Targets.vi"("Function"=enum16{"write", "read"}."read") -> ("Targets"=w293:T50)  [unwired: 5 in, 1 out]
                        n161 = Unbundle(w293) -> ("Target Field (T)"=w292:dbl, "Target Field Rate (T/min)"=w291:dbl)
                      }
                    }
                    n162 = local write "Send to IPS"(w271) -> ()
                    n163 = call-poly <instrlib>:"Signals (Set).vi"("error in"=w288, "Target Field Rate"=w279, "Mercury Reference In"=w286) -> ("error out"=w287:errorcluster, "Mercury Reference Out"=w285:T47)  [unwired: 2 in, 5 out]
                    n164 = local write "Target Field (T) 2"(w278) -> ()
                    n165 = local write "Target Rate (T/min)"(w279) -> ()
                    n166 = Bundle("Target Field (T)"=w278, "Target Field Rate (T/min)"=w279) -> (w281:T51)  [unwired: 1 in]
                    n167 = call-poly <instrlib>:"Signals (Set).vi"("error in"=w287, "Target Field"=w278, "Mercury Reference In"=w285) -> ("error out"=w270:errorcluster)  [unwired: 2 in, 6 out]
                    n168 = call "FGV_PSP - Mercury Actions.vi"("error in"=w270, "Function"=enum16{"write", "read"}."read") -> ("error out"=w275:errorcluster, "Actions"=w273:T49)  [unwired: 4 in]
                    n169 = Bundle By Name(cluster=w273, "Send to IPS"=w271) -> (w277:T49)
                    n170 = call "FGV_PSP - Mercury Actions.vi"("error in"=w275, "Function"=enum16{"write", "read"}."write", "Actions"=w277) -> ("error out"=w272:errorcluster)  [unwired: 3 in, 1 out]
                    n171 = call "FGV_PSP - Mercury Targets.vi"("Function"=enum16{"write", "read"}."write", "Targets"=w281) -> ()  [unwired: 4 in, 2 out]
                  }
                }
              }
              event "Lambda": Value Change {
                # "AUX\nPRES\nHTR\nTEMP"
                n172 = event-data() -> ()  [unwired: 1 in, 6 out]
                n173 = Unbundle By Name(w306) -> ("Mercury ITC Ref"=w305:T52)
                n174 = call-poly <instrlib>:"Open.vi"("error in (no error)"=w304, "Device Identifier"="lambda:LPC", "Mercury Reference In"=w305) -> ("error out"=w301:errorcluster, "Mercury Reference Out"=w300:T47)  [unwired: 7 out]
                n175 = local read "Lambda"() -> (w295:bool)
                n176 = Select(t="ON" ("Sweep Mode"), s=w295, f="OFF" ("Sweep Mode")) -> (s? t:f=w299:string)
                n177 = case shown="False" w295 {
                  frame False {
                    n178 = disable-structure shown="Disabled" {
                      frame Disabled {
                        n179 = property on="Close Needle Valve" class="Bool (strict)"("Val(Sgnl)"=TRUE ("Value (Signaling)")) -> ()  [unwired: 2 in, 2 out]
                      }
                      frame Enabled {
                      }
                    }
                  }
                  frame True {
                  }
                }
                n180 = case shown="False" w295 {
                  frame False {
                    n181 = local write "LPF ON"(timestamp(0 s since 1904-01-01) ("LPF ON")) -> ()
                  }
                  frame True {
                    n182 = Get Date/Time In Seconds() -> (seconds since 1Jan1904=w310:timestamp)
                    n183 = local write "LPF ON"(w310) -> ()
                  }
                }
                n184 = call-poly <instrlib>:"Configuration (Set).vi"("error in"=w301, "Lambda Auto"=w299, "Mercury Reference In"=w300) -> ("error out"=w298:errorcluster, "Response"=w297:T40)  [unwired: 5 in, 2 out]
                n185 = local write "Magnet Status 2"(w297) -> ()
              }
              event "Fast/Slow Fill": Value Change {
                n186 = event-data() -> ()  [unwired: 1 in, 6 out]
                n187 = local read "IPS Devices"() -> (w322:string[])
                n188 = Unbundle By Name(w320) -> ("Mercury IPS Ref"=w325:T47)
                n189 = Index Array(array=w322, index=0) -> (element=w321:string)
                n190 = local read "Fast/Slow Fill"() -> (w318:bool)
                n191 = call-poly <instrlib>:"Open.vi"("error in (no error)"=w324, "Device Identifier"=w321, "Mercury Reference In"=w325) -> ("error out"=w314:errorcluster, "Mercury Reference Out"=w315:T47)  [unwired: 7 out]
                n192 = Select(t="OFF" ("Temperature setpoint"), s=w318, f="ON" ("Temperature setpoint")) -> (s? t:f=w316:string)
                n193 = call-poly <instrlib>:"Configuration (Set).vi"("ISOBUS address"=T39 -1, "error in"=w314, "Delay"=w316, "Mercury Reference In"=w315) -> ("error out"=w311:errorcluster, "Response"=w313:T40)  [unwired: 4 in, 2 out]
                n194 = local write "Magnet Status 2"(w313) -> ()
              }
              event "Close Needle Valve", "Open Needle Valve": Value Change {
                n195 = event-data() -> ()  [unwired: 1 in, 6 out]
                n196 = Unbundle By Name(w339) -> ("Mercury ITC Ref"=w340:T52)
                n197 = Build Array("Close Needle Valve", "Open Needle Valve") -> (w333:bool[])
                n198 = call-poly <instrlib>:"Open.vi"("error in (no error)"=w338, "Device Identifier"="lambda:LPC", "Mercury Reference In"=w340) -> ("error out"=w332:errorcluster, "Mercury Reference Out"=w331:T47)  [unwired: 7 out]
                n199 = Boolean Array To Number(Boolean array=w333) -> (number=w328:u32)
                n200 = case shown="0, Default" w328 {
                  tunnel: w332 -> [w343 w347 w355]
                  tunnel: w331 -> [_ w348 w354]
                  tunnel: [w343 w346 w353] -> w330
                  tunnel: [T40 "" ("Response") w345 w352] -> w329
                  tunnel: [FALSE ("Close Needle Valve") FALSE ("Close Needle Valve") FALSE ("Close Needle Valve")] -> w327
                  frame 0, Default {
                  }
                  frame 1 {
                    n201 = call-poly <instrlib>:"Configuration (Set).vi"("ISOBUS address"=T39 -1, "error in"=w347, "Percentage Open"=0.0, "Mercury Reference In"=w348) -> ("error out"=w346:errorcluster, "Response"=w345:T40)  [unwired: 4 in, 2 out]
                  }
                  frame 2 {
                    n202 = call-poly <instrlib>:"Configuration (Set).vi"("ISOBUS address"=T39 -1, "error in"=w355, "Percentage Open"=100.0, "Mercury Reference In"=w354) -> ("error out"=w353:errorcluster, "Response"=w352:T40)  [unwired: 4 in, 2 out]
                  }
                }
                n203 = local write "Close Needle Valve"(w327) -> ()
                n204 = local write "Open Needle Valve"(w327) -> ()
                n205 = local write "Magnet Status 2"(w329) -> ()
              }
              event "Stop 2": Value Change {
                # "Exit Button Value Change (pressed) Event\n(this executes Macro: Exit to terminate the VI)"
                n206 = event-data() -> ()  [unwired: 1 in, 6 out]
                n207 = call <vilib>:"Add State(s) to Queue__JKI_lib_State_Machine.vi"("State(s) in Front (\"\")"="Macro: Exit", "State(s) in (\"\")"=w362) -> ("States Out"=w361:string)  [unwired: 13 in]
              }
              event "Minimize": Value Change {
                n208 = event-data() -> ()  [unwired: 1 in, 6 out]
              }
              event Panel Close? {
                # "Discard the event because we'll close the front panel ourselves in Macro: Exit"
                # "Close Panel button (pressed) Event\n(this executes Macro: Exit to terminate the VI)"
                n209 = event-data() -> ()  [unwired: 1 in, 1 out]
                n210 = call <vilib>:"Add State(s) to Queue__JKI_lib_State_Machine.vi"("State(s) in Front (\"\")"="Macro: Exit", "State(s) in (\"\")"=w368) -> ("States Out"=w367:string)  [unwired: 13 in]
                n211 = event-data("Discard?"=TRUE) -> ()  [unwired: 1 in, 1 out]
              }
            }
          }
          frame "---------- Core ----------" {
            # "Do not put any code in this frame.\n(it is a separator no-op)"
            n212 = call <vilib>:"Add State(s) to Queue__JKI_lib_State_Machine.vi"("State(s) in (\"\")"=w372) -> ("States Out"=w371:string)  [unwired: 14 in]
          }
          frame Default {
            w382 = 42 items=["No error", "Argument error", "Memory is full", "Out of zone", "End of file", "File already open", "Generic file I/O error", "File not found", "File permission error", "Disk is full", "Duplicate path", "Too many files open", "System feature not enabled", "Resource file not found", "Cannot add resource", "Resource not found", "Image not found", "Image memory error", "Pen does not exist", "Config type invalid", "Config token not found", "Config parse error", "Config memory error", "Bad external code format", "Bad external code offset", "External code not present", "Null window", "Destroy window error", "Null menu", "Print aborted", "Bad print record", "Print driver error", "Windows error during printing", "Memory error during printing", "Print dialog error", "Generic print error", "Invalid device refnum", "Device not found", "Device parameter error", "Device unit error", "Cannot open device", "Device call aborted", "Generic error", "Cancelled by user", "Object ID too low", "Object ID too high", "Object not in heap", "Unknown heap", "Unknown object (invalid DefProc)", "Unknown object (DefProc not in table)", "Message out of range", "Invalid (null) method", "Unknown message", "Manager call not supported", "Bad address", "Network operation in progress", "Network operation timed out", "Connection is busy", "Network attribute not supported", "Network error", "Address in use", "System out of memory", "Connection aborted", "Connection refused", "Not connected", "Already connected", "Connection closed", "Initialization error (interapplication manager)", "Bad occurrence", "Wait on unbound occurrence handler", "Occurrence queue overflow", "Datalog type conflict", "Unused", "Unrecognized type (interapplication manager)", "Memory corrupt", "Failed to make temporary DLL", "Old CIN version", "Drag socket not found", "Failed to load drop-object", "Failed to register OLE object", "Failed to release OLE object", "Format specifier type mismatch", "Unknown format specifier", "Too few format specifiers", "Too many format specifiers", "Scan failed", "Newer CIN version", "Error converting to variant", "Runtime menu error", "Password tampered", "Variant attribute not found", "Incompatible variant data type", "Event data is not available", "Event Store is not present", "Occurrence is not found", "Event Queue is not created", "Event info is not available", "Refnum passed is NULL", "Error retrieving Class GUID", "Error retrieving CoClass GUID", "Error retrieving TypeLib GUID.", "Bad built application magic bytes.", "Specific driver is different from the specific driver associated with the Logical Name.", "There is no session opened to the class driver.", "Max Error", "MAX - Error with config objects", "MAX - Error loading configuration", "MAX - Group not supported"]
            # "Current State"
            # "Do not delete, rename, or modify this frame.\n(this is used to capture unhandled states and typos)"
            # "Handle mistyped state name (developer tool)"
            n213 = Format Into String(format string="Software Exception: Unhandled State \"%s\"." ("message"), error in=w378, w373) -> (resulting string=w381:string, error out=w380:errorcluster)  [unwired: 1 in]
            n214 = call <vilib>:"Error Cluster From Error Code.vi"("show call chain? (False)"=TRUE, "error in (no error)"=w380, "error message (\"\")"=w381, "error code (0)"=w382) -> ("error out"=w379:errorcluster)  [unwired: 5 in]
            n215 = call <vilib>:"Add State(s) to Queue__JKI_lib_State_Machine.vi"("State(s) in (\"\")"=w377) -> ("States Out"=w376:string)  [unwired: 14 in]
          }
          frame "Initialize Core Data" {
            # "Do not delete, rename, or modify this frame.\n(this is used to determine panel behavior on exit)"
            # "originally closed?"
            # "exe?"
            # "If panel starts closed or is an EXE, then close it when we exit"
            n216 = property class="VI"() -> ("Front Panel.Open"=w391:bool)  [unwired: 2 in, 2 out]
            n217 = property class="App"() -> ("App.Kind"=w390:T41)  [unwired: 2 in, 2 out]
            n218 = control-ref of="Current VI Reference"() -> (w384:refnum<vi>)
            n219 = Not(x=w391) -> (.not. x?=w388:bool)
            n220 = Equal?(x=w390, y=T41."Run Time System" ("Application:Kind")) -> (x = y?=w387:bool)
            n221 = Or(x=w388, y=w387) -> (x .or. y?=w385:bool)
            n222 = Bundle By Name(cluster=w386, "Core.Current VI Reference"=w384, "Core.Close Panel on Exit?"=w385) -> (w393:T48)
            n223 = call <vilib>:"Add State(s) to Queue__JKI_lib_State_Machine.vi"("State(s) in (\"\")"=w395) -> ("States Out"=w394:string)  [unwired: 14 in]
          }
          frame "Error Handler" {
            w406 = i32[] [-1950679035, -1950678943]  # Error Codes to Filter
            # "Unhandled Error -- Display it"
            # "Handle any errors here.\nYou can also output any states to clean-up after errors occur"
            # "Clear error"
            n224 = call-poly <userlib>:"Filter Error Codes__ogtk.vi"("Error In"=w407, "Error Codes to Filter"=w406) -> ("Error Out"=w408:errorcluster, "Filtered Error Details"=w405:T53)  [unwired: 7 in, 1 out]
            n225 = Unbundle(w405) -> ("code"=w403:i32, "source"=w404:string)
            n226 = Get Date/Time In Seconds() -> (seconds since 1Jan1904=w402:timestamp)
            n227 = Unbundle By Name(w398) -> ("Error Log"=w400:T34)
            n228 = Bundle By Name(cluster=T42 {"time"=timestamp(0 s since 1904-01-01), "code"=0, "source"=""} ("output cluster"), "time"=w402, "code"=w403, "source"=w404) -> (w399:T42)
            n229 = Build Array (concatenate)(w400, w399) -> (w396:T34)
            "Error List" <- w396
            n230 = Bundle By Name(cluster=w398, "Error Log"=w396) -> (w397:T48)
            n231 = call <vilib>:"General Error Handler.vi"("error in (no error)"=w408) -> ()  [unwired: 10 in, 5 out]
            n232 = call <vilib>:"Add State(s) to Queue__JKI_lib_State_Machine.vi"("State(s) in Front (\"\")"="/* Post Error States", "State(s) in (\"\")"=w412) -> ("States Out"=w411:string)  [unwired: 13 in]
          }
          frame "Exit" {
            # "Do not put any code in this frame.\n(No errors that occur here will be handled.)"
            n233 = call <vilib>:"Add State(s) to Queue__JKI_lib_State_Machine.vi"("State(s) in (\"\")"=w417) -> ("States Out"=w416:string)  [unwired: 14 in]
          }
          frame "---------- Data ----------" {
            # "Do not put any code in this frame.\n(It is a separator no-op. You can make a copy of this frame to create a new Data frame)"
            n234 = call <vilib>:"Add State(s) to Queue__JKI_lib_State_Machine.vi"("State(s) in (\"\")"=w421) -> ("States Out"=w420:string)  [unwired: 14 in]
          }
          frame "Data: Initialize" {
            w422 = T34 []  # Error Log
            w424 = TRUE  # sentinel
            w425 = T47 {"Comms"="", "Device ID"=[], "Comms Layer"=enum."Ethernet TCP/IP", "Command"="", "Query reference"=refnum}  # Mercury IPS Ref
            w426 = T52 {"Comms"="", "Device ID"=[], "Comms Layer"=enum."Ethernet TCP/IP", "Command"="", "Query reference"=refnum}  # Mercury ITC Ref
            w427 = T54 {"Current VI Reference"=refnum, "Close Panel on Exit?"=FALSE}  # Core
            # "do not delete - used by framework"
            # "Expand Bundle to add new data elements to shift register data."
            # "Add new data here."
            # "Data names and types of shift register data are defined by this bundle."
            # "Initialize the shift-register data, here.\n(data names are defined by what you wire into the bundle function)"
            n235 = Bundle("Core"=w427, "Mercury ITC Ref"=w426, "Mercury IPS Ref"=w425, "sentinel"=w424, "Error Log"=w422) -> (w428:T48)  [unwired: 1 in]
            n236 = call <vilib>:"Add State(s) to Queue__JKI_lib_State_Machine.vi"("State(s) in (\"\")"=w430) -> ("States Out"=w429:string)  [unwired: 14 in]
          }
          frame "Data: Cleanup" {
            # "Cleanup any data and references, here.\n(this is called automatically, by the Macro: Exit)"
            n237 = Unbundle By Name(w431) -> ("Core.Current VI Reference"=w434:refnum<vi>)
            n238 = Close Reference(reference=w434, error in (no error)=w433) -> (error out=w432:errorcluster)
            n239 = call <vilib>:"Add State(s) to Queue__JKI_lib_State_Machine.vi"("State(s) in (\"\")"=w436) -> ("States Out"=w435:string)  [unwired: 14 in]
          }
          frame "---------- UI ----------" {
            # "Do not put any code in this frame.\n(It is a separator no-op. You can make a copy of this frame to create a new UI frame)"
            n240 = call <vilib>:"Add State(s) to Queue__JKI_lib_State_Machine.vi"("State(s) in (\"\")"=w440) -> ("States Out"=w439:string)  [unwired: 14 in]
          }
          frame "UI: Initialize" {
            w447 = FALSE
            # "start in local mode"
            # "Initialize the User Interface, here.\n(this is called automatically, by the Macro: Init)"
            n241 = disable-structure shown="Enabled" {
              frame Disabled {
                n242 = Open VI Reference(vi path=path "") -> ()  [unwired: 5 in, 2 out]
                n243 = call "MNK_Dashboard_v2.vi"() -> ()  [unwired: 12 in]
              }
              frame Enabled {
              }
            }
            n244 = Open Application Reference(8:w442) -> (0:w444:errorcluster, 3:w445:refnum<vi>)  [unwired: 3 in]
            n245 = property class="App"(reference=w445, error in=w444, "WebSrvr.Active"=TRUE ("Web Server:Server Active")) -> (error out=w441:errorcluster)  [unwired: 1 out]
            n246 = call <vilib>:"Add State(s) to Queue__JKI_lib_State_Machine.vi"("State(s) in (\"\")"=w452) -> ("States Out"=w451:string)  [unwired: 14 in]
            n247 = local write "Remote Mode"(w447) -> ()
            n248 = call "FGV_PSP - Mercury Remote.vi"("error in"=w441, "Function"=enum16{"write", "read"}."write", "Remote"=w447) -> ("error out"=w446:errorcluster)  [unwired: 3 in, 1 out]
            "Magnet Status 2" <- "" ("Magnet Status 2")
          }
          frame "UI: Cursor Set" {
            # "Argument"
            # "Set and Unset Cursor Busy.\n(Usage: \"UI: Cursor Set >> Busy|Idle\")"
            n249 = case shown="\"Idle\", Default" w454 {
              tunnel: w456 -> [w461 w463]
              tunnel: [w460 w462] -> w455
              frame "Idle", Default {
                n250 = call <vilib>:"Unset Busy.vi"("error in (no error)"=w461) -> ("error out"=w460:errorcluster)  [unwired: 10 in]
              }
              frame "Busy" {
                n251 = call <vilib>:"Set Busy.vi"("error in (no error)"=w463) -> ("error out"=w462:errorcluster)  [unwired: 9 in, 1 out]
              }
            }
            n252 = call <vilib>:"Add State(s) to Queue__JKI_lib_State_Machine.vi"("State(s) in (\"\")"=w459) -> ("States Out"=w458:string)  [unwired: 14 in]
          }
          frame "UI: Front Panel State" {
            # "Argument"
            # "Set Front Panel Open or Closed\n(Usage: \"UI: Front Panel State >> Open|Close\")"
            n253 = Unbundle By Name(w466) -> ("Core.Current VI Reference"=w465:refnum<vi>)
            n254 = case shown="\"Open\", Default" w464 {
              tunnel: w468 -> [w474 w487]
              tunnel: [w476 w488] -> w467
              tunnel: w465 -> [w475 w485]
              frame "Open", Default {
                n255 = property class="VI"(reference=w475, error in=w474) -> (reference out=w472:refnum<vi>, error out=w473:errorcluster, "Front Panel.Open"=w471:bool)
                n256 = case shown="True" w471 {
                  tunnel: [w479 w482] -> w476
                  tunnel: w473 -> [w478 w482]
                  tunnel: w472 -> [w477 _]
                  frame False {
                    n257 = invoke class="VI" method="FP.Open"(reference=w477, error in=w478, "Activate"=TRUE, "State"=T43."Standard") -> (error out=w479:errorcluster)  [unwired: 1 in, 4 out]
                  }
                  frame True {
                  }
                }
              }
              frame "Close" {
                n258 = property class="VI"(reference=w485, error in=w487) -> (reference out=w484:refnum<vi>, error out=w486:errorcluster, "Front Panel.Open"=w483:bool)
                n259 = case shown="True" w483 {
                  tunnel: [w489 w492] -> w488
                  tunnel: w486 -> [w489 w491]
                  tunnel: w484 -> [_ w490]
                  frame False {
                  }
                  frame True {
                    n260 = invoke class="VI" method="FP.Close"(reference=w490, error in=w491) -> (error out=w492:errorcluster)  [unwired: 1 in, 2 out]
                  }
                }
              }
            }
            n261 = call <vilib>:"Add State(s) to Queue__JKI_lib_State_Machine.vi"("State(s) in (\"\")"=w470) -> ("States Out"=w469:string)  [unwired: 14 in]
          }
          frame "---------- Macro ----------" {
            # "Do not put any code in this frame.\n(It is a separator no-op. You can make a copy of this frame to create a new Macro frame)"
            n262 = call <vilib>:"Add State(s) to Queue__JKI_lib_State_Machine.vi"("State(s) in (\"\")"=w496) -> ("States Out"=w495:string)  [unwired: 14 in]
          }
          frame "Macro: Initialize" {
            w497 = "Data: Initialize\nInitialize Core Data\nUI: Initialize\nUI: Front Panel State >> Open\nMercury: Initialize"  # Data: Initialize Initialize Core Data UI: Initialize UI: Front Panel State >> Open Mercury: Initialize
            # "Initialization Macro\n(This is called once, when the VI starts)"
            n263 = call <vilib>:"Add State(s) to Queue__JKI_lib_State_Machine.vi"("State(s) in Front (\"\")"=w497, "State(s) in (\"\")"=w501) -> ("States Out"=w500:string)  [unwired: 13 in]
          }
          frame "Macro: Exit" {
            # "Exit Macro\n(This is called once, when the VI exits)"
            n264 = Unbundle By Name(w514) -> ("Core.Close Panel on Exit?"=w513:bool, "Mercury ITC Ref"=w506:T52, "Mercury IPS Ref"=w505:T47)
            n265 = call <instrlib>:"Close.vi"("error in (no error)"=w504, "Mercury Reference"=w505) -> ("error out"=w503:errorcluster)  [unwired: 9 out]
            n266 = call <instrlib>:"Close.vi"("error in (no error)"=w503, "Mercury Reference"=w506) -> ("error out"=w507:errorcluster)  [unwired: 9 out]
            n267 = call <vilib>:"Simple Error Handler.vi"("error in (no error)"=w507) -> ("error out"=w502:errorcluster)  [unwired: 1 in, 7 out]
            n268 = Select(t="UI: Front Panel State >> Close", s=w513, f="") -> (s? t:f=w510:string)
            n269 = call <vilib>:"Add State(s) to Queue__JKI_lib_State_Machine.vi"("State(s) in (\"\")"=w510, "State(s) at Back (\"\")"="Data: Cleanup\nExit") -> ("States Out"=w508:string)  [unwired: 13 in]
            n270 = call <vilib>:"Add State(s) to Queue__JKI_lib_State_Machine.vi"("State(s) in Front (\"\")"=w508, "State(s) in (\"\")"=w516) -> ("States Out"=w515:string)  [unwired: 13 in]
          }
          frame "---------- New Category ----------" {
            n271 = call <vilib>:"Add State(s) to Queue__JKI_lib_State_Machine.vi"("State(s) in (\"\")"=w520) -> ("States Out"=w519:string)  [unwired: 14 in]
          }
          frame "Mercury: Initialize" {
            w529 = Comms_Transport_Layer."Ethernet TCP/IP" ("Comms Layer")
            n272 = call-poly <instrlib>:"Open.vi"("Clear Previous Connections (False)"=TRUE ("Clear Previous Connections (True)"), "ID Query (True)"=TRUE, "IP Address"="ITC IP Address", "error in (no error)"=w530, "Comms Layer"=w529) -> ("error out"=w523:errorcluster, "# of Instruments"=→"# of Instruments":i32, "Serial Number(s)"=→"Serial Number(s)":string[], "Mercury Reference Out"=w524:T47, "S/W Version(s)"=→"S/W Version(s)":string[])  [unwired: 2 in]
            n273 = call-poly <instrlib>:"Open.vi"("Clear Previous Connections (False)"=FALSE ("Clear Previous Connections (True)"), "ID Query (True)"=TRUE, "IP Address"="IPS IP Address", "error in (no error)"=w523, "Comms Layer"=w529) -> ("error out"=w522:errorcluster, "# of Instruments"=→"# of Instruments 2":i32, "Serial Number(s)"=→"Serial Number(s) 2":string[], "Mercury Reference Out"=w521:T47, "S/W Version(s)"=→"S/W Version(s) 2":string[])  [unwired: 2 in]
            n274 = Bundle By Name(cluster=w538, "Mercury ITC Ref"=w524, "Mercury IPS Ref"=w521) -> (w537:T48)
            n275 = call <vilib>:"Add State(s) to Queue__JKI_lib_State_Machine.vi"("State(s) in (\"\")"=w543, "State(s) at Back (\"\")"="Mercury: Query ITC: System\nMercury: Query IPS: System\nMercury: Query ITC: Temperature\nMercury: Query ITC: Heater\nMercury: Query ITC: Aux\nMercury: Query ITC: Pressure\nMercury: Query IPS: LVL\nMercury: Query IPS: Temperature\nMercury: Query IPS: Magnet" ("State(s) at Back (\"\")")) -> ("States Out"=w542:string)  [unwired: 13 in]
          }
          frame "Mercury: Query ITC: System" {
            n276 = Unbundle By Name(w585) -> ("Mercury ITC Ref"=w545:T52)
            n277 = call-poly <instrlib>:"Configuration (Read).vi"("error in"=w549, "Mercury Reference In"=w545) -> ("error out"=w581:errorcluster, "Devices"=→"ITC Devices":string[], "Mercury Reference Out"=w582:T47)  [unwired: 1 in, 6 out]
            n278 = call-poly <instrlib>:"Configuration (Read).vi"("error in"=w581, "Mercury Reference In"=w582) -> ("error out"=w574:errorcluster, "Automatic Dimming"=→"Automatic Dimming":string, "Mercury Reference Out"=w575:T47)  [unwired: 1 in, 6 out]
            n279 = call-poly <instrlib>:"Configuration (Read).vi"("error in"=w574, "Mercury Reference In"=w575) -> ("error out"=w577:errorcluster, "Dimming Time"=→"Dimming Time":string, "Mercury Reference Out"=w576:T47)  [unwired: 1 in, 6 out]
            n280 = call-poly <instrlib>:"Configuration (Read).vi"("error in"=w577, "Mercury Reference In"=w576) -> ("error out"=w583:errorcluster, "Display Brightness"=→"Display Brightness":string, "Mercury Reference Out"=w584:T47)  [unwired: 1 in, 6 out]
            n281 = call-poly <instrlib>:"Configuration (Read).vi"("error in"=w583, "Mercury Reference In"=w584) -> ("error out"=w568:errorcluster, "Date"=→"Date":string, "Mercury Reference Out"=w567:T47)  [unwired: 1 in, 6 out]
            n282 = call-poly <instrlib>:"Configuration (Read).vi"("error in"=w568, "Mercury Reference In"=w567) -> ("error out"=w570:errorcluster, "Time"=→"Time":string, "Mercury Reference Out"=w569:T47)  [unwired: 1 in, 6 out]
            n283 = call-poly <instrlib>:"Configuration (Read).vi"("error in"=w570, "Mercury Reference In"=w569) -> ("error out"=w548:errorcluster, "time stamp"=→"time stamp":timestamp, "Mercury Reference Out"=w546:T47)  [unwired: 1 in, 6 out]
            n284 = call-poly <instrlib>:"Configuration (Read).vi"("error in"=w548, "Mercury Reference In"=w546) -> ("error out"=w566:errorcluster, "Hardware Version"=→"Hardware Version":string, "Mercury Reference Out"=w565:T47)  [unwired: 1 in, 6 out]
            n285 = call-poly <instrlib>:"Configuration (Read).vi"("error in"=w566, "Mercury Reference In"=w565) -> ("error out"=w564:errorcluster, "Firmware Version"=→"Firmware Version":string, "Mercury Reference Out"=w563:T47)  [unwired: 1 in, 6 out]
            n286 = call-poly <instrlib>:"Configuration (Read).vi"("error in"=w564, "Mercury Reference In"=w563) -> ("error out"=w551:errorcluster, "Serial Number"=→"Serial Number":string, "Mercury Reference Out"=w550:T47)  [unwired: 1 in, 6 out]
            n287 = call-poly <instrlib>:"Configuration (Read).vi"("error in"=w551, "Mercury Reference In"=w550) -> ("error out"=w557:errorcluster, "Free Space"=→"Free Space":i32, "Mercury Reference Out"=w556:T47)  [unwired: 1 in, 6 out]
            n288 = call-poly <instrlib>:"Configuration (Read).vi"("error in"=w557, "Mercury Reference In"=w556) -> ("error out"=w553:errorcluster, "Mode"=→"String":T55, "Mercury Reference Out"=w554:T47)  [unwired: 1 in, 6 out]
            n289 = Get Date/Time In Seconds() -> (seconds since 1Jan1904=w562:timestamp)
            n290 = call-poly <instrlib>:"Configuration (Set).vi"("error in"=w553, "time stamp"=w562, "Mercury Reference In"=w554) -> ("error out"=w547:errorcluster, "Response"=→"Set Date Response":T40)  [unwired: 1 in, 6 out]
            n291 = call <vilib>:"Add State(s) to Queue__JKI_lib_State_Machine.vi"("State(s) in (\"\")"=w587) -> ("States Out"=w586:string)  [unwired: 14 in]
          }
          frame "Mercury: Query ITC: Temperature" {
            # "Temperature"
            n292 = Unbundle By Name(w632) -> ("Mercury ITC Ref"=w589:T52)
            n293 = local read "ITC Devices"() -> (w588:string[])
            n294 = Index Array(array=w588, index=3) -> (element=w590:string)
            n295 = call-poly <instrlib>:"Open.vi"("error in (no error)"=w595, "Device Identifier"=w590, "Mercury Reference In"=w589) -> ("error out"=w607:errorcluster, "Mercury Reference Out"=w608:T47)  [unwired: 7 out]
            n296 = call-poly <instrlib>:"Configuration (Read).vi"("error in"=w607, "Mercury Reference In"=w608) -> ("error out"=w599:errorcluster, "Serial Number"=→"Temp S/N":string, "Mercury Reference Out"=w598:T47)  [unwired: 1 in, 6 out]
            n297 = call-poly <instrlib>:"Configuration (Read).vi"("error in"=w599, "Mercury Reference In"=w598) -> ("error out"=w601:errorcluster, "Nickname"=→"T Nickname":string, "Mercury Reference Out"=w600:T47)  [unwired: 1 in, 6 out]
            n298 = call-poly <instrlib>:"Configuration (Read).vi"("error in"=w601, "Mercury Reference In"=w600) -> ("error out"=w604:errorcluster, "Unit"=→"Unit":T3, "Excitation Magnitude"=→"Excitation Magnitude":dbl, "Mercury Reference Out"=w603:T47)  [unwired: 1 in, 5 out]
            n299 = call-poly <instrlib>:"Configuration (Read).vi"("error in"=w604, "Mercury Reference In"=w603) -> ("error out"=w593:errorcluster, "Sensor Type"=→"Sensor Type":T6, "Mercury Reference Out"=w591:T47)  [unwired: 1 in, 6 out]
            n300 = call-poly <instrlib>:"Configuration (Read).vi"("error in"=w593, "Mercury Reference In"=w591) -> ("error out"=w610:errorcluster, "Excitation Type"=→"Excitation Type":T8, "Mercury Reference Out"=w611:T47)  [unwired: 1 in, 6 out]
            n301 = call-poly <instrlib>:"Configuration (Read).vi"("error in"=w610, "Mercury Reference In"=w611) -> ("error out"=w612:errorcluster, "Unit"=→"H Unit":T3, "Hot Limit"=→"Hot Limit":dbl, "Mercury Reference Out"=w613:T47)  [unwired: 1 in, 5 out]
            n302 = call-poly <instrlib>:"Configuration (Read).vi"("error in"=w612, "Mercury Reference In"=w613) -> ("error out"=w619:errorcluster, "Unit"=→"C Unit":T3, "Cold Limit"=→"Cold Limit":dbl, "Mercury Reference Out"=w618:T47)  [unwired: 1 in, 5 out]
            n303 = call-poly <instrlib>:"Signals (Read).vi"("error in"=w619, "Mercury Reference In"=w618) -> ("error out"=w623:errorcluster, "Unit"=→"V Unit":T3, "Voltage"=→"Voltage":dbl, "Mercury Reference Out"=w622:T47)  [unwired: 1 in, 5 out]
            n304 = call-poly <instrlib>:"Signals (Read).vi"("error in"=w623, "Mercury Reference In"=w622) -> ("error out"=w624:errorcluster, "Unit"=→"T Unit":T3, "Temperature"=→"Temperature":dbl, "Mercury Reference Out"=w627:T47)  [unwired: 1 in, 5 out]
            n305 = call-poly <instrlib>:"Configuration (Read).vi"("error in"=w624, "Mercury Reference In"=w627) -> ("error out"=w630:errorcluster, "Device Details"=→"Temperature Device Settings":T4, "Mercury Reference Out"=w629:T47)  [unwired: 1 in, 6 out]
            n306 = call-poly <instrlib>:"Configuration (Read).vi"("error in"=w630, "Mercury Reference In"=w629) -> ("error out"=w594:errorcluster, "Loop Details"=→"T Loop Details":T11)  [unwired: 1 in, 7 out]
            n307 = call <vilib>:"Add State(s) to Queue__JKI_lib_State_Machine.vi"("State(s) in (\"\")"=w633) -> ("States Out"=w634:string)  [unwired: 14 in]
          }
          frame "Mercury: Query ITC: Heater" {
            # "Heater"
            n308 = Unbundle By Name(w639) -> ("Mercury ITC Ref"=w638:T52)
            n309 = local read "ITC Devices"() -> (w640:string[])
            n310 = Index Array(array=w640, index=2) -> (element=w635:string)
            n311 = call-poly <instrlib>:"Open.vi"("error in (no error)"=w642, "Device Identifier"=w635, "Mercury Reference In"=w638) -> ("error out"=w645:errorcluster, "Mercury Reference Out"=w644:T47)  [unwired: 7 out]
            n312 = call-poly <instrlib>:"Configuration (Read).vi"("error in"=w645, "Mercury Reference In"=w644) -> ("error out"=w652:errorcluster, "Device Details"=→"Heater Device Settings":T13, "Mercury Reference Out"=w651:T47)  [unwired: 1 in, 6 out]
            n313 = call-poly <instrlib>:"Configuration (Read).vi"("error in"=w652, "Mercury Reference In"=w651) -> ("error out"=w654:errorcluster, "Nickname"=→"Htr Nickname":string, "Mercury Reference Out"=w653:T47)  [unwired: 1 in, 6 out]
            n314 = call-poly <instrlib>:"Configuration (Read).vi"("error in"=w654, "Mercury Reference In"=w653) -> ("error out"=w647:errorcluster, "Serial Number"=→"Htr S/N":string, "Mercury Reference Out"=w646:T47)  [unwired: 1 in, 6 out]
            n315 = call-poly <instrlib>:"Configuration (Read).vi"("error in"=w647, "Mercury Reference In"=w646) -> ("error out"=w643:errorcluster, "Unit"=→"Volt Unit":T3, "Voltage Limit"=→"Htr Voltage Limit":dbl, "Mercury Reference Out"=w637:T47)  [unwired: 1 in, 5 out]
            n316 = call-poly <instrlib>:"Configuration (Read).vi"("error in"=w643, "Mercury Reference In"=w637) -> ("error out"=w657:errorcluster, "Unit"=→"Res Unit":T3, "Nominal Resistance"=→"Htr Resistance":dbl, "Mercury Reference Out"=w658:T47)  [unwired: 1 in, 5 out]
            n317 = call-poly <instrlib>:"Configuration (Read).vi"("error in"=w657, "Mercury Reference In"=w658) -> ("error out"=w664:errorcluster, "Unit"=→"Power Unit":T3, "Maximum Power"=→"Maximum Power":dbl, "Mercury Reference Out"=w663:T47)  [unwired: 1 in, 5 out]
            n318 = call-poly <instrlib>:"Signals (Read).vi"("error in"=w664, "Mercury Reference In"=w663) -> ("error out"=w666:errorcluster, "Unit"=→"Htr V Unit":T3, "Voltage"=→"Htr Voltage":dbl, "Mercury Reference Out"=w665:T47)  [unwired: 1 in, 5 out]
            n319 = call-poly <instrlib>:"Signals (Read).vi"("error in"=w666, "Mercury Reference In"=w665) -> ("error out"=w668:errorcluster, "Unit"=→"Htr P Unit":T3, "Power"=→"Htr Power":dbl, "Mercury Reference Out"=w667:T47)  [unwired: 1 in, 5 out]
            n320 = call-poly <instrlib>:"Signals (Read).vi"("error in"=w668, "Mercury Reference In"=w667) -> ("error out"=w636:errorcluster, "Unit"=→"Htr C Unit":T3, "Current"=→"Htr Current":dbl)  [unwired: 1 in, 6 out]
            n321 = call <vilib>:"Add State(s) to Queue__JKI_lib_State_Machine.vi"("State(s) in (\"\")"=w675) -> ("States Out"=w676:string)  [unwired: 14 in]
          }
          frame "Mercury: Query ITC: Aux" {
            # "Auxiliary"
            n322 = Unbundle By Name(w682) -> ("Mercury ITC Ref"=w677:T52)
            n323 = local read "ITC Devices"() -> (w680:string[])
            n324 = Index Array(array=w680, index=0) -> (element=w678:string)
            n325 = call-poly <instrlib>:"Open.vi"("error in (no error)"=w684, "Device Identifier"=w678, "Mercury Reference In"=w677) -> ("error out"=w704:errorcluster, "Mercury Reference Out"=w705:T47)  [unwired: 7 out]
            n326 = call-poly <instrlib>:"Configuration (Read).vi"("error in"=w704, "Mercury Reference In"=w705) -> ("error out"=w708:errorcluster, "Auxiliary Device Details"=→"Auxiliary Device Details":T21, "Mercury Reference Out"=w707:T47)  [unwired: 1 in, 6 out]
            n327 = call-poly <instrlib>:"Configuration (Read).vi"("error in"=w708, "Mercury Reference In"=w707) -> ("error out"=w711:errorcluster, "Serial Number"=→"Aux S/N":string, "Mercury Reference Out"=w710:T47)  [unwired: 1 in, 6 out]
            n328 = call-poly <instrlib>:"Configuration (Read).vi"("error in"=w711, "Mercury Reference In"=w710) -> ("error out"=w713:errorcluster, "Unit"=→"Unit 2":T3, "Min Flow"=→"Min Flow":dbl, "Mercury Reference Out"=w712:T47)  [unwired: 1 in, 5 out]
            n329 = call-poly <instrlib>:"Configuration (Read).vi"("error in"=w713, "Mercury Reference In"=w712) -> ("error out"=w715:errorcluster, "Unit"=→"Unit 3":T3, "Scaling Factor"=→"Scaling Factor":dbl, "Mercury Reference Out"=w714:T47)  [unwired: 1 in, 5 out]
            n330 = call-poly <instrlib>:"Configuration (Read).vi"("error in"=w715, "Mercury Reference In"=w714) -> ("error out"=w683:errorcluster, "Unit"=→"Unit 4":T3, "Temp Err"=→"Temp Err":dbl, "Mercury Reference Out"=w679:T47)  [unwired: 1 in, 5 out]
            n331 = call-poly <instrlib>:"Configuration (Read).vi"("error in"=w683, "Mercury Reference In"=w679) -> ("error out"=w687:errorcluster, "Unit"=→"Unit 5":T3, "Temp V Err"=→"Temp V Err":dbl, "Mercury Reference Out"=w686:T47)  [unwired: 1 in, 5 out]
            n332 = call-poly <instrlib>:"Configuration (Read).vi"("error in"=w687, "Mercury Reference In"=w686) -> ("error out"=w689:errorcluster, "Unit"=→"Unit 6":T3, "Gear"=→"Gear":u32, "Mercury Reference Out"=w688:T47)  [unwired: 1 in, 5 out]
            n333 = call-poly <instrlib>:"Configuration (Read).vi"("error in"=w689, "Mercury Reference In"=w688) -> ("error out"=w697:errorcluster, "Unit"=→"Unit 7":T3, "Speed"=→"Speed":u32, "Mercury Reference Out"=w696:T47)  [unwired: 1 in, 5 out]
            n334 = call-poly <instrlib>:"Signals (Read).vi"("error in"=w697, "Mercury Reference In"=w696) -> ("error out"=w699:errorcluster, "Unit"=→"Unit":T3, "Position"=→"Position":u32, "Mercury Reference Out"=w698:T47)  [unwired: 1 in, 5 out]
            n335 = call-poly <instrlib>:"Signals (Read).vi"("error in"=w699, "Mercury Reference In"=w698) -> ("error out"=w685:errorcluster, "Unit"=→"Unit":T3, "% Open"=→"% Open":dbl)  [unwired: 1 in, 6 out]
            n336 = call <vilib>:"Add State(s) to Queue__JKI_lib_State_Machine.vi"("State(s) in (\"\")"=w722) -> ("States Out"=w723:string)  [unwired: 14 in]
          }
          frame "Mercury: Query ITC: Pressure" {
            # "Pressure"
            n337 = Unbundle By Name(w729) -> ("Mercury ITC Ref"=w726:T52)
            n338 = local read "ITC Devices"() -> (w728:string[])
            n339 = Index Array(array=w728, index=1) -> (element=w725:string)
            n340 = call-poly <instrlib>:"Open.vi"("error in (no error)"=w724, "Device Identifier"=w725, "Mercury Reference In"=w726) -> ("error out"=w732:errorcluster, "Mercury Reference Out"=w733:T47)  [unwired: 7 out]
            n341 = call-poly <instrlib>:"Configuration (Read).vi"("error in"=w732, "Mercury Reference In"=w733) -> ("error out"=w734:errorcluster, "Device Details"=→"Pressure Device":T15, "Mercury Reference Out"=w735:T47)  [unwired: 1 in, 6 out]
            n342 = call-poly <instrlib>:"Configuration (Read).vi"("error in"=w734, "Mercury Reference In"=w735) -> ("error out"=w739:errorcluster, "Nickname"=→"Nickname":string, "Mercury Reference Out"=w740:T47)  [unwired: 1 in, 6 out]
            n343 = call-poly <instrlib>:"Signals (Read).vi"("error in"=w739, "Mercury Reference In"=w740) -> ("error out"=w737:errorcluster, "Current"=→"Current":dbl, "Mercury Reference Out"=w738:T47)  [unwired: 1 in, 6 out]
            n344 = call-poly <instrlib>:"Signals (Read).vi"("error in"=w737, "Mercury Reference In"=w738) -> ("error out"=w730:errorcluster, "Voltage"=→"Voltage":dbl)  [unwired: 1 in, 7 out]
            n345 = call <vilib>:"Add State(s) to Queue__JKI_lib_State_Machine.vi"("State(s) in (\"\")"=w743) -> ("States Out"=w744:string)  [unwired: 14 in]
          }
          frame "Mercury: Query IPS: System" {
            # "Your code here.\n(You can make a copy of, or modify, this frame)"
            n346 = Unbundle By Name(w786) -> ("Mercury IPS Ref"=w747:T47)
            n347 = call-poly <instrlib>:"Configuration (Read).vi"("error in"=w752, "Mercury Reference In"=w747) -> ("error out"=w772:errorcluster, "Devices"=→"IPS Devices":string[], "Mercury Reference Out"=w771:T47)  [unwired: 1 in, 6 out]
            n348 = call-poly <instrlib>:"Configuration (Read).vi"("error in"=w772, "Mercury Reference In"=w771) -> ("error out"=w776:errorcluster, "Automatic Dimming"=→"Automatic Dimming 2":string, "Mercury Reference Out"=w775:T47)  [unwired: 1 in, 6 out]
            n349 = call-poly <instrlib>:"Configuration (Read).vi"("error in"=w776, "Mercury Reference In"=w775) -> ("error out"=w773:errorcluster, "Dimming Time"=→"Dimming Time 2":string, "Mercury Reference Out"=w774:T47)  [unwired: 1 in, 6 out]
            n350 = call-poly <instrlib>:"Configuration (Read).vi"("error in"=w773, "Mercury Reference In"=w774) -> ("error out"=w770:errorcluster, "Display Brightness"=→"Display Brightness 2":string, "Mercury Reference Out"=w769:T47)  [unwired: 1 in, 6 out]
            n351 = call-poly <instrlib>:"Configuration (Read).vi"("error in"=w770, "Mercury Reference In"=w769) -> ("error out"=w779:errorcluster, "Date"=→"Date 2":string, "Mercury Reference Out"=w780:T47)  [unwired: 1 in, 6 out]
            n352 = call-poly <instrlib>:"Configuration (Read).vi"("error in"=w779, "Mercury Reference In"=w780) -> ("error out"=w777:errorcluster, "Time"=→"Time 2":string, "Mercury Reference Out"=w778:T47)  [unwired: 1 in, 6 out]
            n353 = call-poly <instrlib>:"Configuration (Read).vi"("error in"=w777, "Mercury Reference In"=w778) -> ("error out"=w751:errorcluster, "time stamp"=→"time stamp 2":timestamp, "Mercury Reference Out"=w748:T47)  [unwired: 1 in, 6 out]
            n354 = call-poly <instrlib>:"Configuration (Read).vi"("error in"=w751, "Mercury Reference In"=w748) -> ("error out"=w753:errorcluster, "Hardware Version"=→"Hardware Version 2":string, "Mercury Reference Out"=w754:T47)  [unwired: 1 in, 6 out]
            n355 = call-poly <instrlib>:"Configuration (Read).vi"("error in"=w753, "Mercury Reference In"=w754) -> ("error out"=w755:errorcluster, "Firmware Version"=→"Firmware Version 2":string, "Mercury Reference Out"=w756:T47)  [unwired: 1 in, 6 out]
            n356 = call-poly <instrlib>:"Configuration (Read).vi"("error in"=w755, "Mercury Reference In"=w756) -> ("error out"=w761:errorcluster, "Serial Number"=→"Serial Number 2":string, "Mercury Reference Out"=w762:T47)  [unwired: 1 in, 6 out]
            n357 = call-poly <instrlib>:"Configuration (Read).vi"("error in"=w761, "Mercury Reference In"=w762) -> ("error out"=w757:errorcluster, "Free Space"=→"Free Space 2":i32, "Mercury Reference Out"=w758:T47)  [unwired: 1 in, 6 out]
            n358 = call-poly <instrlib>:"Configuration (Read).vi"("error in"=w757, "Mercury Reference In"=w758) -> ("error out"=w760:errorcluster, "Mode"=→"String 2":T55, "Mercury Reference Out"=w759:T47)  [unwired: 1 in, 6 out]
            n359 = Get Date/Time In Seconds() -> (seconds since 1Jan1904=w768:timestamp)
            n360 = call-poly <instrlib>:"Configuration (Set).vi"("error in"=w760, "time stamp"=w768, "Mercury Reference In"=w759) -> ("error out"=w750:errorcluster, "Response"=→"Set Date Response 2":T40)  [unwired: 1 in, 6 out]
            n361 = call <vilib>:"Add State(s) to Queue__JKI_lib_State_Machine.vi"("State(s) in (\"\")"=w788) -> ("States Out"=w787:string)  [unwired: 14 in]
          }
          frame "Mercury: Query IPS: LVL" {
            # "Level"
            n362 = Unbundle By Name(w828) -> ("Mercury IPS Ref"=w791:T47)
            n363 = local read "IPS Devices"() -> (w827:string[])
            n364 = Index Array(array=w827, index=0) -> (element=w790:string)
            n365 = call-poly <instrlib>:"Open.vi"("error in (no error)"=w797, "Device Identifier"=w790, "Mercury Reference In"=w791) -> ("error out"=w813:errorcluster, "Mercury Reference Out"=w812:T47)  [unwired: 7 out]
            n366 = call-poly <instrlib>:"Configuration (Read).vi"("error in"=w813, "Mercury Reference In"=w812) -> ("error out"=w818:errorcluster, "LVL Device Settings"=→"LVL Device DetailSettings":T23, "Mercury Reference Out"=w815:T47)  [unwired: 1 in, 6 out]
            n367 = call-poly <instrlib>:"Configuration (Read).vi"("error in"=w818, "Mercury Reference In"=w815) -> ("error out"=w819:errorcluster, "Serial Number"=→"LVL S/N":string, "Mercury Reference Out"=w817:T47)  [unwired: 1 in, 6 out]
            n368 = call-poly <instrlib>:"Configuration (Read).vi"("error in"=w819, "Mercury Reference In"=w817) -> ("error out"=w822:errorcluster, "Resistance Configuration"=→"He Res Config":T28, "Mercury Reference Out"=w821:T47)  [unwired: 1 in, 6 out]
            n369 = call-poly <instrlib>:"Configuration (Read).vi"("error in"=w822, "Mercury Reference In"=w821) -> ("error out"=w824:errorcluster, "Magnitude"=→"LVL P Magnitude":dbl, "Mercury Reference Out"=w823:T47)  [unwired: 1 in, 6 out]
            n370 = call-poly <instrlib>:"Configuration (Read).vi"("error in"=w824, "Mercury Reference In"=w823) -> ("error out"=w796:errorcluster, "Duration"=→"LVL P Duration":dbl, "Mercury Reference Out"=w794:T47)  [unwired: 1 in, 6 out]
            n371 = call-poly <instrlib>:"Configuration (Read).vi"("error in"=w796, "Mercury Reference In"=w794) -> ("error out"=w800:errorcluster, "Freq 100%"=→"N Freq 100%":dbl, "Mercury Reference Out"=w799:T47)  [unwired: 1 in, 6 out]
            n372 = call-poly <instrlib>:"Configuration (Read).vi"("error in"=w800, "Mercury Reference In"=w799) -> ("error out"=w803:errorcluster, "Pulse Period"=→"N Pulse Period":dbl, "Mercury Reference Out"=w802:T47)  [unwired: 1 in, 6 out]
            n373 = call-poly <instrlib>:"Signals (Read).vi"("error in"=w803, "Mercury Reference In"=w802) -> ("error out"=w805:errorcluster, "Resistance"=→"He Resistance":dbl, "Mercury Reference Out"=w804:T47)  [unwired: 1 in, 6 out]
            n374 = call-poly <instrlib>:"Signals (Read).vi"("error in"=w805, "Mercury Reference In"=w804) -> ("error out"=w807:errorcluster, "Level"=→"He Level" →"He LEVEL":dbl, "Mercury Reference Out"=w806:T47)  [unwired: 1 in, 6 out]
            n375 = call-poly <instrlib>:"Signals (Read).vi"("error in"=w807, "Mercury Reference In"=w806) -> ("error out"=w809:errorcluster, "Counter"=→"N Counter":u32, "Mercury Reference Out"=w808:T47)  [unwired: 1 in, 6 out]
            n376 = call-poly <instrlib>:"Signals (Read).vi"("error in"=w809, "Mercury Reference In"=w808) -> ("error out"=w795:errorcluster, "Level"=→"N Level" →"N2 LEVEL":dbl)  [unwired: 1 in, 7 out]
            n377 = call <vilib>:"Add State(s) to Queue__JKI_lib_State_Machine.vi"("State(s) in (\"\")"=w829) -> ("States Out"=w830:string)  [unwired: 14 in]
          }
          frame "Mercury: Query IPS: Temperature" {
            n378 = Unbundle By Name(w875) -> ("Mercury IPS Ref"=w832:T47)
            n379 = local read "IPS Devices"() -> (w874:string[])
            n380 = Index Array(array=w874, index=4) -> (element=w833:string)
            n381 = call-poly <instrlib>:"Open.vi"("error in (no error)"=w831, "Device Identifier"=w833, "Mercury Reference In"=w832) -> ("error out"=w862:errorcluster, "Mercury Reference Out"=w857:T47)  [unwired: 7 out]
            n382 = call-poly <instrlib>:"Configuration (Read).vi"("error in"=w862, "Mercury Reference In"=w857) -> ("error out"=w863:errorcluster, "Serial Number"=→"Temp S/N 2":string, "Mercury Reference Out"=w858:T47)  [unwired: 1 in, 6 out]
            n383 = call-poly <instrlib>:"Configuration (Read).vi"("error in"=w863, "Mercury Reference In"=w858) -> ("error out"=w864:errorcluster, "Nickname"=→"T Nickname 2":string, "Mercury Reference Out"=w859:T47)  [unwired: 1 in, 6 out]
            n384 = call-poly <instrlib>:"Configuration (Read).vi"("error in"=w864, "Mercury Reference In"=w859) -> ("error out"=w865:errorcluster, "Unit"=→"Unit 12":T3, "Excitation Magnitude"=→"Excitation Magnitude 2":dbl, "Mercury Reference Out"=w860:T47)  [unwired: 1 in, 5 out]
            n385 = call-poly <instrlib>:"Configuration (Read).vi"("error in"=w865, "Mercury Reference In"=w860) -> ("error out"=w866:errorcluster, "Sensor Type"=→"Sensor Type 2":T6, "Mercury Reference Out"=w861:T47)  [unwired: 1 in, 6 out]
            n386 = call-poly <instrlib>:"Configuration (Read).vi"("error in"=w866, "Mercury Reference In"=w861) -> ("error out"=w836:errorcluster, "Excitation Type"=→"Excitation Type 2":T8, "Mercury Reference Out"=w835:T47)  [unwired: 1 in, 6 out]
            n387 = call-poly <instrlib>:"Configuration (Read).vi"("error in"=w836, "Mercury Reference In"=w835) -> ("error out"=w842:errorcluster, "Unit"=→"H Unit 2":T3, "Hot Limit"=→"Hot Limit 2":dbl, "Mercury Reference Out"=w837:T47)  [unwired: 1 in, 5 out]
            n388 = call-poly <instrlib>:"Configuration (Read).vi"("error in"=w842, "Mercury Reference In"=w837) -> ("error out"=w843:errorcluster, "Unit"=→"C Unit 2":T3, "Cold Limit"=→"Cold Limit 2":dbl, "Mercury Reference Out"=w838:T47)  [unwired: 1 in, 5 out]
            n389 = call-poly <instrlib>:"Signals (Read).vi"("error in"=w843, "Mercury Reference In"=w838) -> ("error out"=w844:errorcluster, "Unit"=→"V Unit 2":T3, "Voltage"=→"Voltage 2":dbl, "Mercury Reference Out"=w839:T47)  [unwired: 1 in, 5 out]
            n390 = call-poly <instrlib>:"Signals (Read).vi"("error in"=w844, "Mercury Reference In"=w839) -> ("error out"=w845:errorcluster, "Unit"=→"T Unit 2":T3, "Temperature"=→"Temperature 2":dbl, "Mercury Reference Out"=w840:T47)  [unwired: 1 in, 5 out]
            n391 = call-poly <instrlib>:"Configuration (Read).vi"("error in"=w845, "Mercury Reference In"=w840) -> ("error out"=w846:errorcluster, "Device Details"=→"Temperature Device Settings 2":T4, "Mercury Reference Out"=w841:T47)  [unwired: 1 in, 6 out]
            n392 = call-poly <instrlib>:"Configuration (Read).vi"("error in"=w846, "Mercury Reference In"=w841) -> ("error out"=w834:errorcluster, "Loop Details"=→"T Loop Details 2":T11)  [unwired: 1 in, 7 out]
            n393 = call <vilib>:"Add State(s) to Queue__JKI_lib_State_Machine.vi"("State(s) in (\"\")"=w876) -> ("States Out"=w877:string)  [unwired: 14 in]
          }
          frame "Mercury: Query IPS: Magnet" {
            n394 = Unbundle By Name(w916) -> ("Mercury IPS Ref"=w882:T47)
            n395 = call-poly <instrlib>:"Open.vi"("error in (no error)"=w878, "Device Identifier"="Device Identifier", "Mercury Reference In"=w882) -> ("error out"=w901:errorcluster, "Mercury Reference Out"=w900:T47)  [unwired: 7 out]
            n396 = call-poly <instrlib>:"Configuration (Read).vi"("error in"=w901, "Mercury Reference In"=w900) -> ("error out"=w904:errorcluster, "Magnet Device Details"=→"Magnet Device Details":T31, "Mercury Reference Out"=w903:T47)  [unwired: 1 in, 6 out]
            n397 = call-poly <instrlib>:"Configuration (Read).vi"("error in"=w904, "Mercury Reference In"=w903) -> ("error out"=w907:errorcluster, "Serial Number"=→"Mag S/N":string, "Mercury Reference Out"=w906:T47)  [unwired: 1 in, 6 out]
            n398 = call-poly <instrlib>:"Configuration (Read).vi"("error in"=w907, "Mercury Reference In"=w906) -> ("error out"=w910:errorcluster, "Bipolar Output"=→"Bipolar Output":string, "Mercury Reference Out"=w909:T47)  [unwired: 1 in, 6 out]
            n399 = call-poly <instrlib>:"Configuration (Read).vi"("error in"=w910, "Mercury Reference In"=w909) -> ("error out"=w913:errorcluster, "Out Config"=→"Out Config":T56, "Mercury Reference Out"=w912:T47)  [unwired: 1 in, 6 out]
            n400 = call-poly <instrlib>:"Configuration (Read).vi"("error in"=w913, "Mercury Reference In"=w912) -> ("error out"=w884:errorcluster, "Unit"=→"Unit 8":T3, "Current Limit"=→"Current Limit":dbl, "Mercury Reference Out"=w881:T47)  [unwired: 1 in, 5 out]
            n401 = call-poly <instrlib>:"Configuration (Read).vi"("error in"=w884, "Mercury Reference In"=w881) -> ("error out"=w887:errorcluster, "Unit"=→"Unit 9":T3, "AtoB"=→"AtoB":dbl, "Mercury Reference Out"=w886:T47)  [unwired: 1 in, 5 out]
            n402 = call-poly <instrlib>:"Configuration (Read).vi"("error in"=w887, "Mercury Reference In"=w886) -> ("error out"=w890:errorcluster, "Switch Present"=→"Switch Present":string, "Mercury Reference Out"=w889:T47)  [unwired: 1 in, 6 out]
            n403 = call-poly <instrlib>:"Configuration (Read).vi"("error in"=w890, "Mercury Reference In"=w889) -> ("error out"=w895:errorcluster, "Unit"=→"Unit 10":T3, "SW VLIM"=→"SW VLIM":dbl, "Mercury Reference Out"=w894:T47)  [unwired: 1 in, 5 out]
            n404 = call-poly <instrlib>:"Signals (Read).vi"("error in"=w895, "Mercury Reference In"=w894) -> ("error out"=w897:errorcluster, "Unit"=→"Unit 11":T3, "Current Rate"=→"Current Rate":dbl, "Mercury Reference Out"=w896:T47)  [unwired: 1 in, 5 out]
            n405 = call-poly <instrlib>:"Signals (Read).vi"("error in"=w897, "Mercury Reference In"=w896) -> ("error out"=w883:errorcluster, "PSU Act Stat"=→"PSU Act Stat":T37)  [unwired: 1 in, 7 out]
            n406 = call <vilib>:"Add State(s) to Queue__JKI_lib_State_Machine.vi"("State(s) in (\"\")"=w917) -> ("States Out"=w918:string)  [unwired: 14 in]
          }
          frame "Mercury: IPS: Idle - 1" {
            n407 = Unbundle By Name(w959) -> ("Mercury IPS Ref"=w927:T47)
            n408 = local read "Device Identifier"() -> (w940:T33)
            n409 = call-poly <instrlib>:"Configuration (Read).vi"("error in"=w958, "Mercury Reference In"=w927) -> ("error out"=w947:errorcluster, "Time"=w951:string, "Mercury Reference Out"=w948:T47)  [unwired: 1 in, 6 out]
            n410 = local write "Time 2"(w951) -> ()
            n411 = call-poly <instrlib>:"Open.vi"("error in (no error)"=w947, "Device Identifier"=w940, "Mercury Reference In"=w948) -> ("error out"=w946:errorcluster, "Mercury Reference Out"=w945:T47)  [unwired: 7 out]
            n412 = call-poly <instrlib>:"Signals (Read).vi"("error in"=w946, "Mercury Reference In"=w945) -> ("error out"=w957:errorcluster, "Switch Heater Status"=w949:string, "Mercury Reference Out"=w954:T47)  [unwired: 1 in, 6 out]
            n413 = Equal?(x=w949, y="ON") -> (x = y?=w924:bool)
            "SWITCH HEATER" <- w924
            n414 = call-poly <instrlib>:"Signals (Read).vi"("error in"=w957, "Mercury Reference In"=w954) -> ("error out"=w956:errorcluster, "Current"=→"Current (A)" →"Current (A)":dbl, "Mercury Reference Out"=w953:T47)  [unwired: 1 in, 6 out]
            n415 = call-poly <instrlib>:"Signals (Read).vi"("error in"=w956, "Mercury Reference In"=w953) -> ("error out"=w939:errorcluster, "Voltage"=→"Voltage (V) 2" →"Voltage (V)":dbl, "Mercury Reference Out"=w938:T47)  [unwired: 1 in, 6 out]
            n416 = call-poly <instrlib>:"Signals (Read).vi"("error in"=w939, "Mercury Reference In"=w938) -> ("error out"=w941:errorcluster, "Field"=→"Power Supply Field (T)":dbl, "Mercury Reference Out"=w944:T47)  [unwired: 1 in, 6 out]
            n417 = call-poly <instrlib>:"Signals (Read).vi"("error in"=w941, "Mercury Reference In"=w944) -> ("error out"=w942:errorcluster, "Target Field Rate"=→"Target  Rate (T/min)":dbl, "Mercury Reference Out"=w943:T47)  [unwired: 1 in, 6 out]
            n418 = call-poly <instrlib>:"Signals (Read).vi"("error in"=w942, "Mercury Reference In"=w943) -> ("error out"=w937:errorcluster, "Target Field"=→"Target Field (T)":dbl, "Mercury Reference Out"=w936:T47)  [unwired: 1 in, 6 out]
            n419 = call-poly <instrlib>:"Signals (Read).vi"("error in"=w937, "Mercury Reference In"=w936) -> ("error out"=w955:errorcluster, "Persistant Field"=→"Magnet Field (T)" →"Magnet Field (T) 2":dbl, "Mercury Reference Out"=w952:T47)  [unwired: 1 in, 6 out]
            n420 = call-poly <instrlib>:"Signals (Read).vi"("error in"=w955, "Mercury Reference In"=w952) -> ("error out"=w921:errorcluster, "PSU Act Stat"=w928:T37)  [unwired: 1 in, 7 out]
            n421 = call "FGV_PSP - Mercury Status.vi"("error in"=w921, "Function"=enum16{"write", "read"}."read") -> ("error out"=w923:errorcluster, "Status"=w920:T57)  [unwired: 4 in]
            n422 = local write "PSU Act Stat"(w928) -> ()
            n423 = Bundle By Name(cluster=w920, "Switch"=w924) -> (w919:T57)
            n424 = case shown="\"CLMP\"" w928 {
              selector: w928 -> [w962 _ _ _ _]
              tunnel: [w962 "Holding" "Ramping to Setpoint" "Ramping to Zero" "Clamped"] -> w935
              frame Default {
              }
              frame "HOLD" {
              }
              frame "RTOS" {
              }
              frame "RTOZ" {
              }
              frame "CLMP" {
              }
            }
            "Magnet Status 3" <- w935
            n425 = call "FGV_PSP - Mercury Status.vi"("error in"=w923, "Function"=enum16{"write", "read"}."write", "Status"=w919) -> ("error out"=w922:errorcluster)  [unwired: 3 in, 1 out]
            n426 = call <vilib>:"Add State(s) to Queue__JKI_lib_State_Machine.vi"("State(s) in (\"\")"=w960) -> ("States Out"=w961:string)  [unwired: 14 in]
          }
          frame "Mercury: IPS: Idle - 2" {
            n427 = Unbundle By Name(w1019) -> ("Mercury IPS Ref"=w987:T47)
            n428 = local read "IPS Devices"() -> (w1013:string[])
            n429 = Index Array(array=w1013, index=0) -> (element=w1012:string)
            n430 = call-poly <instrlib>:"Open.vi"("error in (no error)"=w999, "Device Identifier"=w1012, "Mercury Reference In"=w987) -> ("error out"=w1015:errorcluster, "Mercury Reference Out"=w1016:T47)  [unwired: 7 out]
            n431 = call-poly <instrlib>:"Signals (Read).vi"("error in"=w1015, "Mercury Reference In"=w1016) -> ("error out"=w1017:errorcluster, "Level"=w967:dbl, "Mercury Reference Out"=w1018:T47)  [unwired: 1 in, 6 out]
            "He LVL Chart" <- w967
            "He LEVEL 3" <- w967
            n432 = Greater?(x=w967, y=20.0) -> (0:w996:bool)
            n433 = Greater?(x=w967, y=50.0) -> (0:w997:bool)
            n434 = call-poly <instrlib>:"Signals (Read).vi"("error in"=w1017, "Mercury Reference In"=w1018) -> ("error out"=w1002:errorcluster, "Level"=w988:dbl)  [unwired: 1 in, 7 out]
            "N2 LVL Chart" <- w988
            n435 = case shown="False" w996 {
              tunnel: [w1027 u32 6618880] -> w985
              tunnel: w997 -> [w1028 _]
              frame False {
                n436 = case shown="False" w1028 {
                  tunnel: [u32 16711680 u32 16776704] -> w1027
                  frame False {
                  }
                  frame True {
                  }
                }
              }
              frame True {
              }
            }
            n437 = local write "He LEVEL"(w967) -> ()
            n438 = local read "IPS Devices"() -> (w1007:string[])
            n439 = property on="He LVL Chart" class="Slide (strict)"("Fill Color"=w985) -> ()  [unwired: 2 in, 2 out]
            n440 = property on="He LEVEL 3" class="DigNum (strict)"("NumText.TextColor"=w985) -> ()  [unwired: 2 in, 2 out]
            n441 = local write "N2 LEVEL"(w988) -> ()
            n442 = Index Array(array=w1007, index=5) -> (element=w1005:string)
            n443 = local read "Target  Rate (T/min)"() -> (w977:dbl)
            n444 = local read "Power Supply Field (T)"() -> (w975:dbl)
            n445 = call-poly <instrlib>:"Open.vi"("error in (no error)"=w1002, "Device Identifier"=w1005, "Mercury Reference In"=w987) -> ("error out"=w1004:errorcluster, "Mercury Reference Out"=w1003:T47)  [unwired: 7 out]
            n446 = local read "Magnet Field (T) 2"() -> (w974:dbl)
            n447 = Greater?(x=w988, y=20.0) -> (0:w990:bool)
            n448 = Greater?(x=w988, y=50.0) -> (0:w989:bool)
            n449 = local read "Target Field (T)"() -> (w976:dbl)
            n450 = local read "Current (A)"() -> (w979:dbl)
            n451 = local read "Voltage (V)"() -> (w978:dbl)
            n452 = case shown="False" w990 {
              tunnel: [w1022 u32 6618880] -> w986
              tunnel: w989 -> [w1023 _]
              frame False {
                n453 = case shown="False" w1023 {
                  tunnel: [u32 16711680 u32 16776704] -> w1022
                  frame False {
                  }
                  frame True {
                  }
                }
              }
              frame True {
              }
            }
            n454 = call-poly <instrlib>:"Signals (Read).vi"("error in"=w1004, "Mercury Reference In"=w1003) -> ("error out"=w972:errorcluster, "Temperature"=w969:dbl, "Mercury Reference Out"=w970:T47)  [unwired: 1 in, 6 out]
            "Magnet T" <- w969
            n455 = call-poly <instrlib>:"Signals (Read).vi"("error in"=w972, "Mercury Reference In"=w970) -> ("error out"=w971:errorcluster, "Resistance"=w968:dbl)  [unwired: 1 in, 7 out]
            "Magnet R" <- w968
            n456 = property on="N2 LVL Chart" class="Slide (strict)"("Fill Color"=w986) -> ()  [unwired: 2 in, 2 out]
            n457 = property on="N2 LEVEL" class="DigNum (strict)"("NumText.TextColor"=w986) -> ()  [unwired: 2 in, 2 out]
            n458 = local read "PSU Act Stat"() -> (w995:string)
            n459 = call "FGV_PSP - Mercury Status.vi"("error in"=w971, "Function"=enum16{"write", "read"}."read") -> ("error out"=w982:errorcluster, "Status"=w980:T57)  [unwired: 4 in]
            n460 = Bundle By Name(cluster=w980, "Magnet Field"=w974, "PS Field"=w975, "Target Field"=w976, "Target Field Rate"=w977, "Voltage"=w978, "Current"=w979) -> (w981:T57)
            n461 = call "FGV_PSP - Mercury Status.vi"("error in"=w982, "Function"=enum16{"write", "read"}."write", "Status"=w981) -> ("error out"=w1000:errorcluster)  [unwired: 3 in, 1 out]
            n462 = Bundle(cluster=T44 {"Magnet Field"=0.0, "PS Field"=0.0, "Target Field"=0.0, "Target Field Rate"=0.0, "Voltage"=0.0, "Current"=0.0}, "Magnet Field"=w974, "PS Field"=w975, "Target Field"=w976, "Target Field Rate"=w977, "Voltage"=w978, "Current"=w979) -> (w984:T44)
            n463 = call "FGV_PSP - Mercury Action Status.vi"("error in"=w1000, "Function"=enum16{"write", "read"}."write", "Mercury Status"=w995) -> ("error out"=w998:errorcluster)  [unwired: 3 in, 1 out]
            n464 = Cluster To Array(cluster=w984) -> (array=w1009:dbl[])
            n465 = Build Array(w995) -> (w1001:string[])
            n466 = Build Array (concatenate)(w1009, w988, w967, w969, w968) -> (w1008:dbl[])
            n467 = call "1820_IPS_to_DSC.vi"("str"=w1001, "dbl"=w1008) -> ()  [unwired: 2 in]
            n468 = call <vilib>:"Add State(s) to Queue__JKI_lib_State_Machine.vi"("State(s) in (\"\")"=w1020) -> ("States Out"=w1021:string)  [unwired: 14 in]
          }
          frame "Mercury: ITC: Idle" {
            n469 = Unbundle By Name(w1061) -> ("Mercury ITC Ref"=w1042:T52)
            n470 = local read "ITC Devices"() -> (w1057:string[])
            n471 = Index Array(array=w1057, index=3) -> (element=w1056:string)
            n472 = call-poly <instrlib>:"Open.vi"("error in (no error)"=w1037, "Device Identifier"=w1056, "Mercury Reference In"=w1042) -> ("error out"=w1055:errorcluster, "Mercury Reference Out"=w1049:T47)  [unwired: 7 out]
            n473 = call-poly <instrlib>:"Signals (Read).vi"("error in"=w1055, "Mercury Reference In"=w1049) -> ("error out"=w1035:errorcluster, "Temperature"=w1040:dbl, "Mercury Reference Out"=w1034:T47)  [unwired: 1 in, 6 out]
            "LPF T" <- w1040
            n474 = call-poly <instrlib>:"Signals (Read).vi"("error in"=w1035, "Mercury Reference In"=w1034) -> ("error out"=w1033:errorcluster, "Resistance"=w1032:dbl)  [unwired: 1 in, 7 out]
            "LPF R" <- w1032
            n475 = local read "ITC Devices"() -> (w1060:string[])
            n476 = Index Array(array=w1060, index=1) -> (element=w1058:string)
            n477 = call-poly <instrlib>:"Open.vi"("error in (no error)"=w1033, "Device Identifier"=w1058, "Mercury Reference In"=w1042) -> ("error out"=w1054:errorcluster, "Mercury Reference Out"=w1053:T47)  [unwired: 7 out]
            n478 = call-poly <instrlib>:"Configuration (Read).vi"("error in"=w1054, "Mercury Reference In"=w1053) -> ("error out"=w1048:errorcluster, "Device Details"=w1052:T15)  [unwired: 1 in, 7 out]
            n479 = local read "ITC Devices"() -> (w1046:string[])
            n480 = Unbundle By Name(w1052) -> ("Pressure Signals.Pressure"=w1051:string)
            n481 = Index Array(array=w1046, index=0) -> (element=w1045:string)
            n482 = call-poly <instrlib>:"Open.vi"("error in (no error)"=w1048, "Device Identifier"=w1045, "Mercury Reference In"=w1042) -> ("error out"=w1044:errorcluster, "Mercury Reference Out"=w1043:T47)  [unwired: 7 out]
            n483 = Fract/Exp String To Number(string=w1051) -> (number=w1039:dbl)  [unwired: 3 in, 1 out]
            "LPF Pressure" <- w1039
            n484 = call-poly <instrlib>:"Signals (Read).vi"("error in"=w1044, "Mercury Reference In"=w1043) -> ("error out"=w1036:errorcluster, "% Open"=w1038:dbl)  [unwired: 1 in, 7 out]
            "LPF NV (%)" <- w1038
            n485 = Build Array(w1040, w1039, w1038, w1032) -> (w1041:dbl[])
            n486 = call "1820_ITC_to_DSC.vi"("dbl"=w1041) -> ()  [unwired: 3 in]
            n487 = call <vilib>:"Add State(s) to Queue__JKI_lib_State_Machine.vi"("State(s) in (\"\")"=w1062) -> ("States Out"=w1063:string)  [unwired: 14 in]
          }
          frame "Mercury: Empty" {
            n488 = Unbundle By Name(w1065) -> ()  [unwired: 1 out]
            n489 = call <vilib>:"Add State(s) to Queue__JKI_lib_State_Machine.vi"("State(s) in (\"\")"=w1066) -> ("States Out"=w1067:string)  [unwired: 14 in]
          }
          frame "Mercury: IPS: Idle - 3" {
            n490 = call "Oxford_MNK_Omega_Sign.vi"("error in (no error)"=w1069) -> ("error out"=w1068:errorcluster)  [unwired: 10 in]
            n491 = call <vilib>:"Add State(s) to Queue__JKI_lib_State_Machine.vi"("State(s) in (\"\")"=w1071) -> ("States Out"=w1072:string)  [unwired: 14 in]
          }
        }
      }
      n492 = disable-structure shown="Disabled" {
        frame Disabled {
          (unwired) FALSE
          n493 = call-poly <instrlib>:"Configuration (Read).vi"() -> ()  [unwired: 3 in, 9 out]
          n494 = disable-structure shown="Disabled" {
            frame Disabled {
              n495 = property on="Fast/Slow Fill" class="Bool (strict)" props=["Val(Sgnl)"]() -> ()  [unwired: 3 in, 2 out]
            }
            frame Enabled {
            }
          }
          n496 = local read "PS Heat"() -> ()  [unwired: 1 in]
          n497 = local read "Lambda"() -> ()  [unwired: 1 in]
          n498 = local write "PS Heat"(FALSE) -> ()
          n499 = local read "Clamp"() -> ()  [unwired: 1 out]
        }
        frame Enabled {
        }
      }
    }
    frame Enabled {
    }
  }
